vi "Measurement.vi"(0 "Position":T7(array[cluster]) {"Z" format="%.1f"; "Y" format="%.1f"; "X" format="%.1f"}, 1 "setup":T8=enum."Show Setup", 2 "Post Process":T5, 4 "File":T9, 5 "Results file":path, 7 "Raw data file":path, 11 "Setup filename":string) -> (14 "2nd plot":cluster{"Xo":dbl, "Delta X":dbl, dbl[]}[](graph), 19 "Status Out":T4)   [LabVIEW 2011]
uses:
  Anemometry Sub Vis/Controls/Save_Data.ctl
  Anemometry Sub Vis/Controls/Setup.ctl
  Anemometry Sub Vis/Controls/Graph_Type.ctl
  Anemometry Sub Vis/Controls/Post_Process.ctl
  Anemometry Sub Vis/Gen Trav/Multi_Run_Status.ctl
  Anemometry Sub Vis/Controls/Board_Types.ctl
  Anemometry Sub Vis/File/Setup_Filetype.ctl
  Anemometry Sub Vis/Controls/Block_start_and_end.ctl
  ADAM Client/Sub VIs/ADAM Controls/Traverse_Level_State.ctl
  Anemometry Sub Vis/Globals/Trav_pos_global.vi
  Anemometry Sub Vis/Globals/Meas_global.vi
  Anemometry Sub Vis/Acquisition/Data_Translation/DataTranslation_global.vi
  Anemometry Sub Vis/Acquisition/PWA/PWAtasksGLOBAL.vi
  Anemometry Sub Vis/Globals/Preference_global.vi
  Anemometry Sub Vis/Globals/LDA_meas_global_1.vi
  Anemometry Sub Vis/Globals/Dynamic_call_global.ph.vi
  Anemometry Sub Vis/Globals/LDA_meas_global_2.vi
  Anemometry Sub Vis/Globals/Plug_in_data_global.vi
panel:
  in  "PP next block":bool
  out "Pause message":string
  out "Statistics":string[][](table)
  in  "Tab Control":T1(tab)
  out "Measurement time (min)":dbl=6.0 format="%.2f"
  in  "No of bins":i32=80
  in  "Show Smoth":bool=TRUE
  in  "Second Graph":T3={"Plot 1"=2, "Plot 2"=1, "Save graph"=0, "Plot Type"=enum."Vel histogram"} {"Save graph" items=["Do not save plot", "Save plot"]; "Plot 2" items=["Nothing", "Mano (Pitot)", "RV (Uhw)", "RV (Kulite)"]; "Plot 1" items=["Nothing", "Mano (Pitot)", "RV (Uhw)", "RV (Kulite)"]}
  in  "First Graph":T3={"Plot 1"=1, "Plot 2"=2, "Save graph"=0, "Plot Type"=enum."Velocity trace"} {"Save graph" items=["Do not save plot", "Save plot"]; "Plot 2" items=["Nothing", "Mano (Pitot)", "RV (Uhw)", "RV (Kulite)"]; "Plot 1" items=["Nothing", "Mano (Pitot)", "RV (Uhw)", "RV (Kulite)"]}
  out "First plot":cluster{"Xo":dbl, "Delta X":dbl, dbl[]}[](graph)
  in  "Comments":string
  out "BSA Diagnostic info":string[][](table)
  out "uv":dbl[][](graph)=[[-0.041806189081711534, -0.046435429052714985, -0.04035660097427599, -0.042187605126076694, -0.042052555599004206]]
  out "u^4":dbl[][](graph)
  out "u^3":dbl[][](graph)
  out "u^2":dbl[][](graph)=[[0.09743628875280319, 0.10575821456272283, 0.10126262927293661, 0.09890442087602569, 0.1022948212436432]]
  out "U":dbl[][](graph)=[[0.8295029456391334, 0.8915896983798417, 0.8415763502225625, 0.8394746126219594, 0.8466062785395404]]
  in  "Block average display control":cluster{"Name":string, "Include":bool}[](array[cluster])=[{"Name"="FF (C)", "Include"=FALSE}]
  out "Array U":dbl[][](array[numeric]) format="%.2e"
  out "Array u^2":dbl[][](array[numeric]) format="%.2e"
  out "Actual Sampling freq":dbl=100.0 format="%.1f"
  in  "Desired Sampling freq (Hz)":dbl=100.0 format="%.1f"
  in  "Correlate?":T6(ring)
  out "Current Block No":i32=5
  in  "Pause":bool
  in  "No of Blocks":i32=5
  in  "stop":bool
  in  "No of samples":i32=1000 min=0 step=1
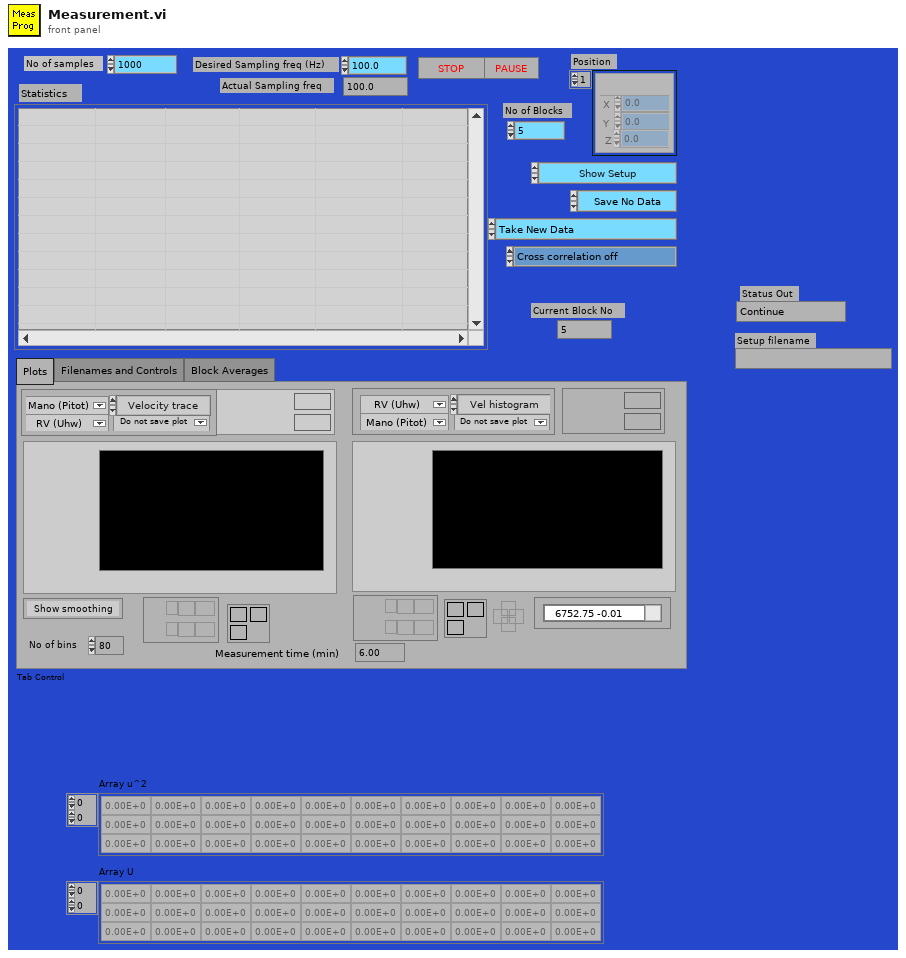
[diagram p1: front panel]
types:
  T1 = enum32{"Plots", "Filenames and Controls", "Block Averages"}
  T2 = typedef "Graph_Type.ctl" = enum16{"Show no graph", "Voltage trace", "Velocity trace", "Vel histogram", "Spectrum", "f.E(f) v Log f", "Auto-Corr"}
  T3 = cluster{"Plot 1":u16, "Plot 2":u16, "Save graph":u16, "Plot Type":T2}
  T4 = typedef "Multi_Run_Status.ctl" = enum16{"Continue", "Jump to Next Point", "Jump to Next Row", "Jump To Fall Back", "Terminate Run"}
  T5 = typedef "Post_Process.ctl" = enum16{"Take New Data", "Post Process Raw Data File"}
  T6 = enum16{"Cross correlation off", "Show correlation panel", "Correlate without activating panel"}
  T7 = cluster{"Name":string, "X":dbl, "Y":dbl, "Z":dbl}[]
  T8 = typedef "Setup.ctl" = enum16{"Run Program", "Show Setup", "Save Current Setup", "Setup Front Panel"}
  T9 = typedef "Save_Data.ctl" = enum16{"Save No Data", "Save Data"}
  T10 = enum32{"Bad", "Idle", "Run top level", "Running"}
  T11 = enum16{"Velocity", "Transit time", "Arrival time"}
  T12 = enum16{"Save no data", "Save data in new files", "Save data in existing files"}
  T13 = typedef "Board_Types.ctl" = enum16{"Simulate", "Local ADAM", "Server ADAM", "NI-DAQmx", "NI-DAQmxBase", "ADC488", "DT LV-link"}
  T14 = typedef "Setup_Filetype.ctl" = enum16{"Measurement Setups", "Calibration Setups", "General", "Results File Plotter Setups", "Speed Calib Tweaks"}
  T15 = typedef "Block_start_and_end.ctl" = cluster{"Started":dbl, "Ended":dbl, "Analogue Frequency Hz":dbl}
  T16 = typedef "Traverse_Level_State.ctl" = enum16{"Running", "Complete"}
  T17 = typedef "Traverse_cluster.ctl" = cluster{"Start X":dbl, "Start Y":dbl, "Start Z":dbl, "End X":dbl, "End Y":dbl, "End Z":dbl, "No. of pts.":i32, "Spacing":T18, "Filename":path, "Tunnel Speed":dbl, "Averaging time (min)":dbl, "Extra Commands":string, "Specific Arguments":string, "Emission Rate (l/min)":dbl, "Trace Gas Concentration (%)":dbl, "Density Ratio":string, "Comments":string, "Row No":i32, "Row Type Selector":T19, "Completion time":string, "Row Duration (mins)":dbl, "No. of Valid pts.":i32, "Meas Setup File":string}
  T18 = typedef "Spacing.ctl" = enum16{"Linear", "Log", "Gauss", "Specified", "N/A"}
  T19 = typedef "Multi_run_mode.ctl" = enum16{"Move Traverse Only", "Set Tunnel Speed Only", "Set Source Only", "Set Measurement Conditions", "Single Measurement", "Vertical Profile", "Lateral Profile", "Longitudinal Profile", "Explore Volume", "Multi-Axis Profile", "Auto Calibrate", "Meas Fast FID Bkgnd", "Check Beam Power", "Scanning Valve Measurement", "Run VI Named:", "Set ADAM Ch", "Wait (minutes)", "Send Message", "Synchronize With:", "Fall Back to this Row", "Turn Off Row Repeating", "Blank Row"}
  T20 = typedef "Analysis_info_cluster.ctl" = cluster{"Colour":u32, "Inst type":T21, "Inst name":string, "Symbol":string, "Code name":string, "Extra Info":string, "Inst Array":T22, "Index":i32, "Voltage Index":i32, "Extra Titles":string[], "Extra Values":string[]}
  T21 = typedef "Inst_type.ctl" = enum16{"Propeller anemometer", "Raw voltage", "Pressure Transducer", "Pitot-static tube", "Preston tube", "Hot wire", "Cross wire 1", "Cross wire 2", "Generic Linear", "Generic Polynomial", "Generic BackPoly", "Fast FID", "Thermocouple", "Cold wire", "Pulsed Wire", "LDA Vel", "LDA Tran time", "LDA Arr time"}
  T22 = typedef "Instrument_Array.ctl" = enum16{"PWA", "LDA", "Analogue"}
  T23 = enum16{"Velocity", "Transit time", "Arrival time"}[]
  T24 = typedef "BSA_Type.ctl" = enum16{"57N11", "BSA F60"}
  T25 = typedef "BSA_info_Cluster.ctl" = cluster{"GPIB Address":string, "No of Check Bytes":i32, "Extra Info":string, "COLOUR":u32, "Wavelength (nm)":dbl}
  T26 = typedef "Ch_and_Spans.ctl" = cluster{"high limit (10V)":sgl, "low limit (-10V)":sgl, "Ch No":i16, "Var name":string, "Use Latest Calib":bool}
  T27 = typedef "Velocity_cluster.ctl" = cluster{"Name":string, "U":dbl, "u^2":dbl, "u^3/(u^2)^(1.5)":dbl, "u^4/(u^2)^2 -3":dbl, "% u'/U":dbl, "Mean % Err":dbl, "u^4":dbl}
  T28 = typedef "Analysis_type_cluster.ctl" = cluster{"Analysis type":T29, "Indicies":i32[], "Name":string, "Inst Array":T22, "Info index":i32}
  T29 = typedef "Analysis_type_Enum.ctl" = enum16{"Slow Response", "Fast Response", "Weighted Fast Response", "Fast FID", "Weighted Fast FID", "Cross Wire", "Weighted Cross Wire", "Weighted LDA"}
  T30 = cluster{"Insts for plotting[0]":u16, "Insts for plotting[1]":u16}
  T31 = typedef "PWA_Data.ctl" = enum16{"No PWA Data", "One Ch PWA"}
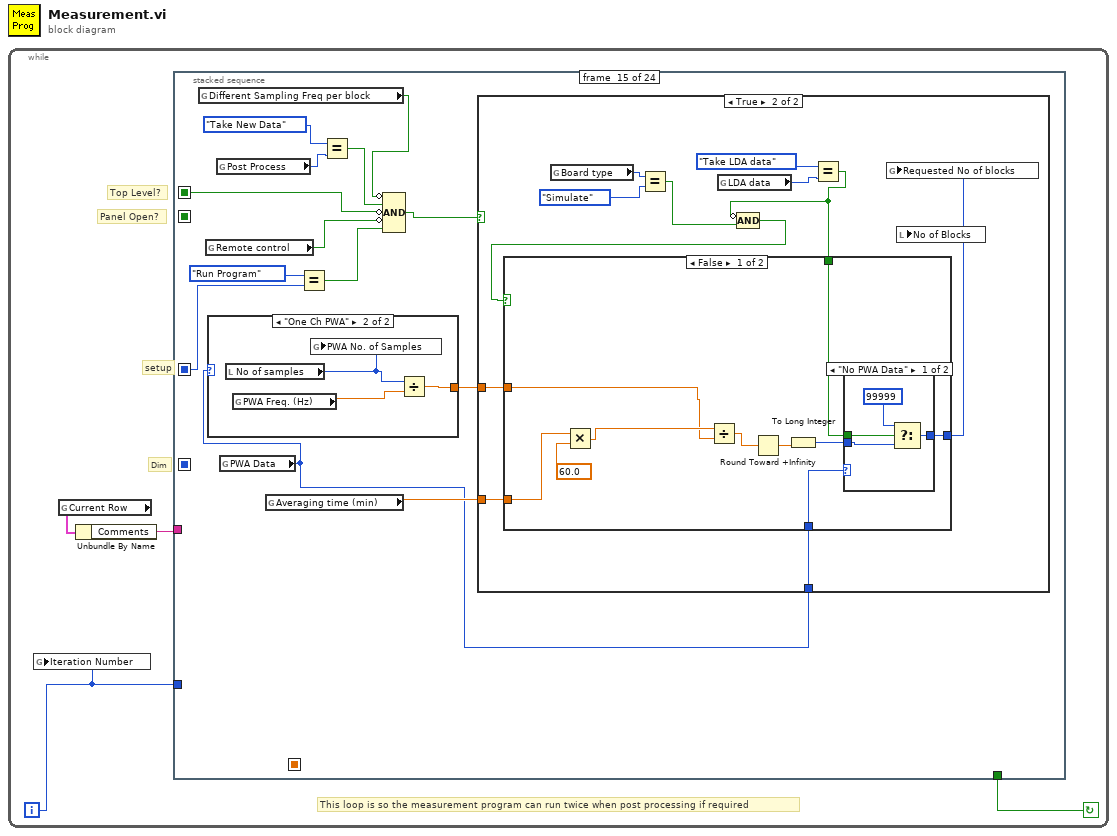
[diagram p0: block diagram]
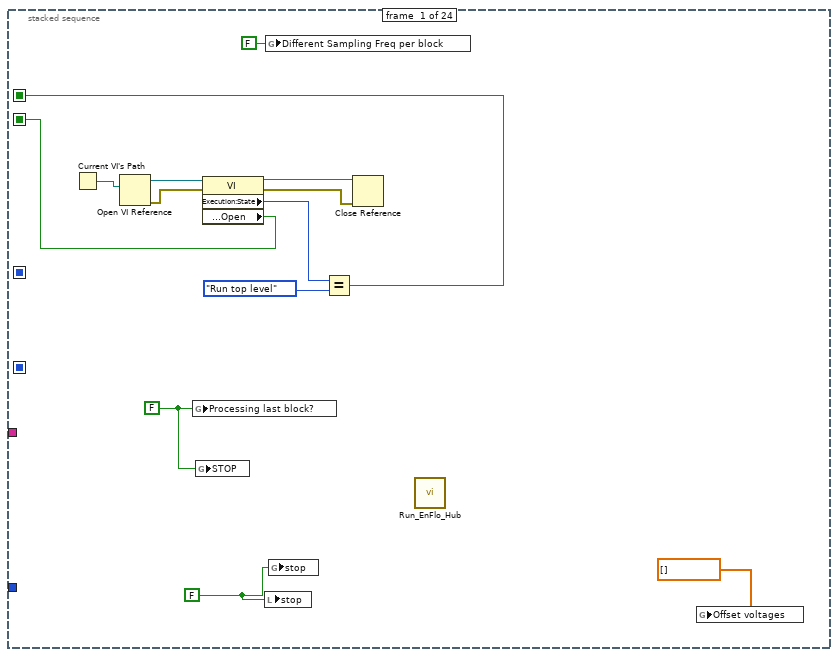
[diagram p2: hidden frame]
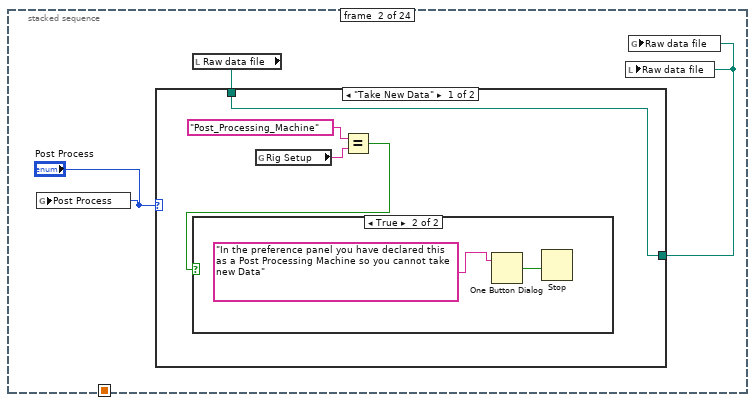
[diagram p3: hidden frame]
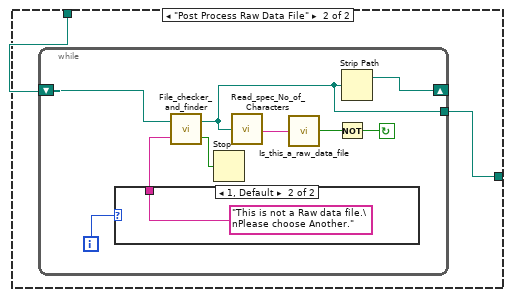
[diagram p5: hidden frame]
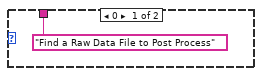
[diagram p6: hidden frame]
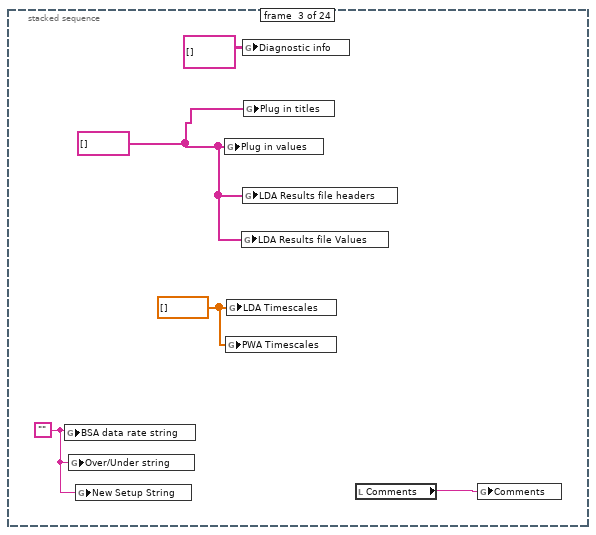
[diagram p7: hidden frame]
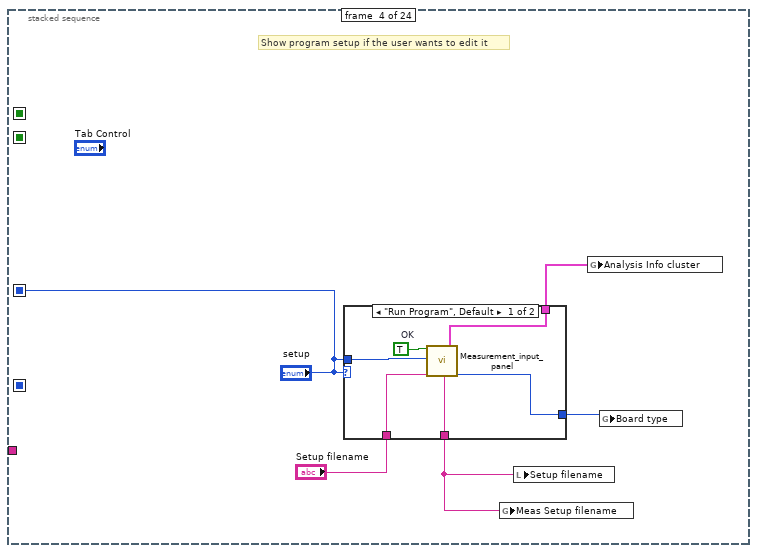
[diagram p8: hidden frame]
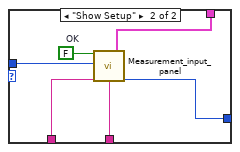
[diagram p9: hidden frame]
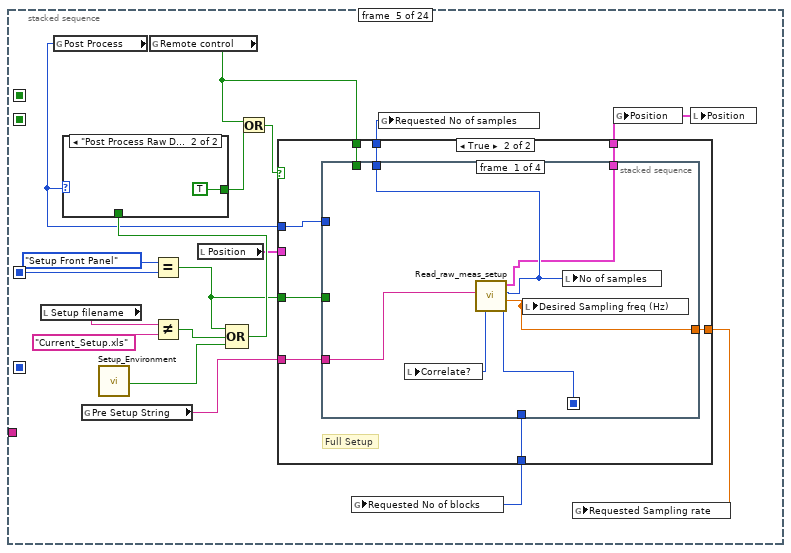
[diagram p10: hidden frame]
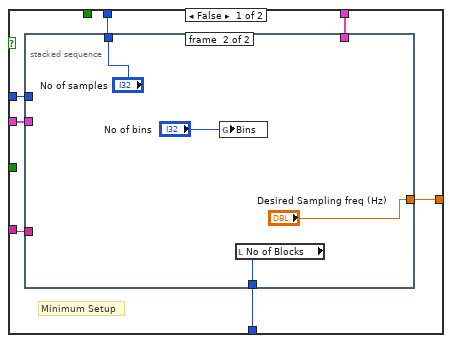
[diagram p12: hidden frame]
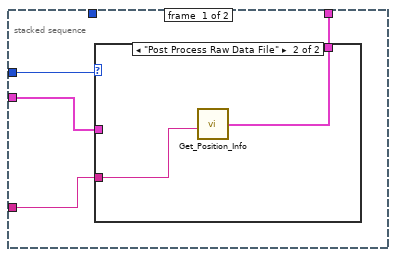
[diagram p13: hidden frame]
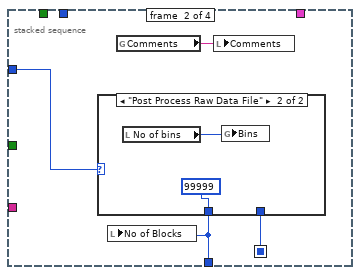
[diagram p15: hidden frame]
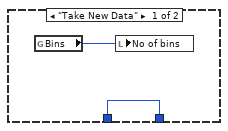
[diagram p16: hidden frame]
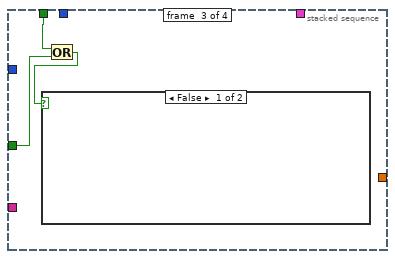
[diagram p17: hidden frame]
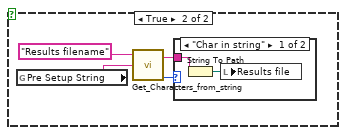
[diagram p18: hidden frame]
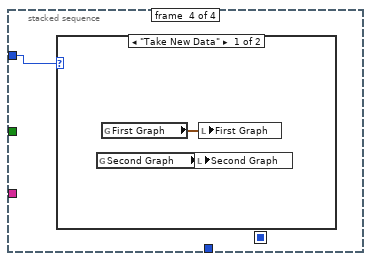
[diagram p20: hidden frame]
diagram:
  n1 = while {
    i -> [w1]
    stop <- w2 continue-if-true
    # "This loop is so the measurement program can run twice when post processing if required"
    # "Panel Open?"
    # "Top Level?"
    # "setup"
    # "Dim"
    n2 = global write "Meas_global.vi" "Iteration Number"(w1) -> ()
    n3 = global read "Trav_pos_global.vi" "Current Row"() -> (w3:T17)
    n4 = Unbundle By Name(w3) -> ("Comments"=w4:string)
    n5 = stacked-sequence {
      seq-local: [_ _ _ _ _ _ _ _ w187 _ _ _ _ _ _ _ _ _ _ _ _ _ _ _] -> [_ _ _ _ _ _ _ _ _ _ _ _ _ _ _ _ _ w626 _ _ _ _ _ _]
      seq-local: [_ _ _ "setup" _ _ _ _ _ _ _ _ _ _ _ _ _ _ _ _ _ _ _ _] -> [_ _ _ _ w71 _ _ _ w179 w264 _ _ _ _ w524 w564 w571 w627 w935 w1011 w1039 _ _ w1114]
      seq-local: [_ _ _ _ _ _ _ _ _ _ _ _ _ _ _ _ w567 _ _ _ _ _ _ _] -> [_ _ _ _ _ _ _ _ _ _ _ _ _ _ _ _ _ w625 w918 _ _ _ _ _]
      seq-local: [w7 _ _ _ _ _ _ _ _ _ _ _ _ _ _ _ _ _ _ _ _ _ _ _] -> [_ _ _ _ _ _ _ _ _ w244 _ _ _ _ w520 _ _ w624 _ _ _ _ _ _]
      seq-local: [w6 _ _ _ _ _ _ _ _ _ _ _ _ _ _ _ _ _ _ _ _ _ _ _] -> [_ _ _ _ _ _ _ _ _ _ _ _ w363 _ _ _ _ _ _ _ _ _ _ _]
      tunnel: w4 -> [_ _ _ _ _ _ _ w172 _ _ _ _ _ _ _ _ _ _ _ _ _ _ w1082 _]
      tunnel: w1 -> [_ _ _ _ _ _ _ _ _ _ _ _ _ _ _ _ _ _ _ _ _ _ w1077 _]
      tunnel: [_ _ _ _ _ _ _ _ _ _ _ _ _ _ _ _ _ _ _ _ _ _ w1076 _] -> w2
      frame #0 {
        w15 = FALSE ("Processing last block?")
        w16 = FALSE ("stop")
        n6 = Current VI's Path() -> (path=w8:path)
        n7 = Open VI Reference(vi path=w8) -> (vi reference=w9:refnum<vi>, error out=w10:errorcluster)  [unwired: 1 in, 4 out]
        n8 = global write "Meas_global.vi" "Processing last block?"(w15) -> ()
        n9 = global write "PWAtasksGLOBAL.vi" "STOP"(w15) -> ()
        n10 = property class="VI"(reference=w9, error in=w10) -> (reference out=w11:refnum<vi>, error out=w12:errorcluster, "Execution:State"=w13:T10, "Front Panel.Open"=w6:bool)
        n11 = local write "stop"(w16) -> ()
        n12 = global write "DataTranslation_global.vi" "Different Sampling Freq per block"(FALSE ("Different Sampling Freq per block")) -> ()
        n13 = global write "Meas_global.vi" "stop"(w16) -> ()
        n14 = Equal?(x=w13, y=T10."Run top level" ("Exec.State")) -> (x = y?=w7:bool)
        n15 = Close Reference(reference=w11, error in (no error)=w12) -> ()  [unwired: 1 out]
        n16 = call "Run_EnFlo_Hub.vi"() -> ()  [unwired: 8 out]
        n17 = global write "Meas_global.vi" "Offset voltages"(dbl[] [] ("Offset voltages used")) -> ()
      }
      frame #1 {
        n18 = global write "Meas_global.vi" "Post Process"("Post Process") -> ()
        n19 = local read "Raw data file"() -> (w20:path)
        n20 = case shown="\"Take New Data\"" "Post Process" {
          tunnel: [w24 w28] -> w19
          tunnel: w20 -> [w24 w27]
          frame "Take New Data" {
            n21 = global read "Preference_global.vi" "Rig Setup"() -> (w23:string)
            n22 = Equal?(x="Post_Processing_Machine" ("Rig Setup"), y=w23) -> (x = y?=w21:bool)
            n23 = case shown="True" w21 {
              frame False {
              }
              frame True {
                n24 = One Button Dialog(message="In the preference panel you have declared this as a Post Processing Machine so you cannot take new Data") -> (true=w25:bool)  [unwired: 1 in]
                n25 = Stop(stop? (T)=w25) -> ()
              }
            }
          }
          frame "Post Process Raw Data File" {
            n26 = while {
              tunnel: [w30] -> w28
              shift-left: w27 -> [w32]
              shift-right: [w31] -> _
              i -> [w33]
              stop <- w34 continue-if-true
              n27 = case shown="1, Default" w33 {
                tunnel: ["Find a Raw Data File to Post Process" ("Promp if not found") "This is not a Raw data file.\nPlease choose Another." ("Promp if not found")] -> w37
                frame 0 {
                }
                frame 1, Default {
                }
              }
              n28 = call "File_checker_and_finder.vi"("Promp if not found"=w37, "Filename In"=w32) -> ("cancelled"=w29:bool, "Filename Out"=w30:path)
              n29 = Stop(stop? (T)=w29) -> ()
              n30 = call "Read_spec_No_of_Characters.vi"("Filename"=w30) -> ("character string"=w36:string)  [unwired: 1 out]
              n31 = call "Is_this_a_raw_data_file.vi"("character string"=w36) -> ("Raw Dat File?"=w35:bool)  [unwired: 2 out]
              n32 = Not(x=w35) -> (.not. x?=w34:bool)
              n33 = Strip Path(path=w30) -> (stripped path=w31:path)  [unwired: 1 out]
            }
          }
        }
        n34 = local write "Raw data file"(w19) -> ()
        n35 = global write "Meas_global.vi" "Raw data file"(w19) -> ()
      }
      frame #2 {
        w42 = dbl[] [] ("LDA Timescales")
        w41 = string[] [] ("Plug in values")
        w44 = ""
        n36 = global write "Meas_global.vi" "BSA data rate string"(w44) -> ()
        n37 = global write "Meas_global.vi" "Over/Under string"(w44) -> ()
        n38 = global write "Meas_global.vi" "New Setup String"(w44) -> ()
        n39 = global write "Dynamic_call_global.ph.vi" "Plug in values"(w41) -> ()
        n40 = global write "PWAtasksGLOBAL.vi" "PWA Timescales"(w42) -> ()
        n41 = global write "LDA_meas_global_1.vi" "LDA Timescales"(w42) -> ()
        n42 = global write "LDA_meas_global_1.vi" "LDA Results file Values"(w41) -> ()
        n43 = global write "Meas_global.vi" "Diagnostic info"(string[][] [] ("Diagnostic info")) -> ()
        n44 = global write "LDA_meas_global_1.vi" "LDA Results file headers"(w41) -> ()
        n45 = global write "Dynamic_call_global.ph.vi" "Plug in titles"(w41) -> ()
        n46 = local read "Comments"() -> (w43:string)
        n47 = global write "Meas_global.vi" "Comments"(w43) -> ()
      }
      frame #3 {
        # "Show program setup if the user wants to edit it"
        n48 = case shown="\"Run Program\", Default" "setup" {
          tunnel: [w54 w60] -> w49
          tunnel: [w53 w59] -> w48
          tunnel: "Setup filename" -> [w52 w58]
          tunnel: [w51 w57] -> w45
          tunnel: "setup" -> [w50 w56]
          frame "Run Program", Default {
            w55 = TRUE  # OK
            n49 = call "Measurement_input_panel.vi"("OK"=w55, "setup"=w50, "Setup filename"=w52) -> ("Setup filename out"=w51:string, "Analysis Info cluster"=w54:T20[], "Board type"=w53:T13)  [unwired: 14 out]
          }
          frame "Show Setup" {
            w61 = FALSE  # OK
            n50 = call "Measurement_input_panel.vi"("OK"=w61, "setup"=w56, "Setup filename"=w58) -> ("Setup filename out"=w57:string, "Analysis Info cluster"=w60:T20[], "Board type"=w59:T13)  [unwired: 14 out]
          }
        }
        n51 = global write "Meas_global.vi" "Meas Setup filename"(w45) -> ()
        n52 = local write "Setup filename"(w45) -> ()
        n53 = global write "Meas_global.vi" "Analysis Info cluster"(w49) -> ()
        n54 = global write "Meas_global.vi" "Board type"(w48) -> ()
      }
      frame #4 {
        n55 = local read "Setup filename"() -> (w75:string)
        n56 = global read "Meas_global.vi" "Post Process"() -> (w70:T5)
        n57 = global read "Meas_global.vi" "Pre Setup String"() -> (w66:string)
        n58 = call "Setup_Environment.vi"() -> ("First Time"=w67:bool)  [unwired: 1 in]
        n59 = global read "Meas_global.vi" "Remote control"() -> (w63:bool)
        n60 = Equal?(x=Setup."Setup Front Panel" ("setup"), y=w71) -> (x = y?=w62:bool)
        n61 = Not Equal?(x=w75, y="Current_Setup.xls" ("Setup filename")) -> (x != y?=w73:bool)
        n62 = local read "Position"() -> (w64:T7)
        n63 = Compound Arithmetic op=OR(w62, w73, w67) -> (w72:bool)
        n64 = case shown="\"Post Process Raw Data File\"" w70 {
          tunnel: [w80 TRUE] -> w79
          tunnel: w72 -> [w80 _]
          frame "Take New Data" {
          }
          frame "Post Process Raw Data File" {
          }
        }
        n65 = Or(x=w63, y=w79) -> (x .or. y?=w78:bool)
        n66 = case shown="True" w78 {
          tunnel: w70 -> [w84 w107]
          tunnel: [w88 w106] -> w68
          tunnel: [w87 w101] -> w77
          tunnel: [w86 w105] -> w76
          tunnel: [w85 w104] -> w65
          tunnel: w66 -> [w83 w103]
          tunnel: w64 -> [w82 _]
          tunnel: w63 -> [_ w102]
          tunnel: w62 -> [_ w100]
          frame False {
            # "Minimum Setup"
            n67 = stacked-sequence {
              tunnel: [_ "Desired Sampling freq (Hz)"] -> w88
              tunnel: [_ w98] -> w87
              tunnel: [_ "No of samples"] -> w86
              tunnel: [w91 _] -> w85
              tunnel: w84 -> [w92 _]
              tunnel: w83 -> [w90 _]
              tunnel: w82 -> [w89 _]
              frame #0 {
                n68 = case shown="\"Post Process Raw Data File\"" w92 {
                  tunnel: [w93 w94] -> w91
                  tunnel: w89 -> [w93 _]
                  tunnel: w90 -> [_ w95]
                  frame "Take New Data" {
                  }
                  frame "Post Process Raw Data File" {
                    n69 = call "Get_Position_Info.vi"("Input string"=w95) -> ("Position"=w94:T7)
                  }
                }
              }
              frame #1 {
                n70 = global write "Meas_global.vi" "Bins"("No of bins") -> ()
                n71 = local read "No of Blocks"() -> (w98:i32)
              }
            }
          }
          frame True {
            # "Full Setup"
            n72 = stacked-sequence {
              seq-local: [w110 _ _ _] -> [_ w115 _ _]
              tunnel: w107 -> [_ w116 _ w131]
              tunnel: [w113 _ _ _] -> w106
              tunnel: [w112 _ _ _] -> w105
              tunnel: [w108 _ _ _] -> w104
              tunnel: w103 -> [w111 _ _ _]
              tunnel: w102 -> [_ _ w124 _]
              tunnel: [_ w114 _ _] -> w101
              tunnel: w100 -> [_ _ w123 _]
              frame #0 {
                n73 = call "Read_raw_meas_setup.vi"("Setup file string"=w111) -> ("No of Blocks"=w110:i32, "Sampling freq (Hz)"=w113:dbl, "No of samples"=w112:i32, "Position"=w108:T7, "Correlate?"=w109:T6)  [unwired: 4 out]
                n74 = local write "Correlate?"(w109) -> ()
                n75 = local write "Desired Sampling freq (Hz)"(w113) -> ()
                n76 = local write "No of samples"(w112) -> ()
              }
              frame #1 {
                n77 = case shown="\"Post Process Raw Data File\"" w116 {
                  tunnel: [w119 99999 ("No of Blocks")] -> w114
                  tunnel: w115 -> [w119 _]
                  frame "Take New Data" {
                    n78 = global read "Meas_global.vi" "Bins"() -> (w118:i32)
                    n79 = local write "No of bins"(w118) -> ()
                  }
                  frame "Post Process Raw Data File" {
                    n80 = local read "No of bins"() -> (w120:i32)
                    n81 = global write "Meas_global.vi" "Bins"(w120) -> ()
                  }
                }
                n82 = local write "No of Blocks"(w114) -> ()
                n83 = global read "Meas_global.vi" "Comments"() -> (w117:string)
                n84 = local write "Comments"(w117) -> ()
              }
              frame #2 {
                n85 = Or(x=w124, y=w123) -> (x .or. y?=w122:bool)
                n86 = case shown="False" w122 {
                  frame False {
                  }
                  frame True {
                    n87 = global read "Meas_global.vi" "Pre Setup String"() -> (w125:string)
                    n88 = call "Get_Characters_from_string.vi"("Input string"=w125, "Variable name"="Results filename") -> ("Status"=w128:enum16{"Char in string", "Char not in string"}, "Value"=w127:string)  [unwired: 1 in]
                    n89 = case shown="\"Char in string\"" w128 {
                      tunnel: w127 -> [w130 _]
                      frame "Char in string" {
                        n90 = String To Path(string=w130) -> (path=w129:path)
                        n91 = local write "Results file"(w129) -> ()
                      }
                      frame "Char not in string" {
                      }
                    }
                  }
                }
              }
              frame #3 {
                n92 = case shown="\"Take New Data\"" w131 {
                  frame "Take New Data" {
                    n93 = global read "Meas_global.vi" "Second Graph"() -> (w132:T3)
                    n94 = global read "Meas_global.vi" "First Graph"() -> (w133:T3)
                    n95 = local write "Second Graph"(w132) -> ()
                    n96 = local write "First Graph"(w133) -> ()
                  }
                  frame "Post Process Raw Data File" {
                  }
                }
              }
            }
          }
        }
        n97 = global write "Meas_global.vi" "Requested No of blocks"(w77) -> ()
        n98 = global write "Meas_global.vi" "Requested No of samples"(w76) -> ()
        n99 = global write "Meas_global.vi" "Requested Sampling rate"(w68) -> ()
        n100 = global write "Meas_global.vi" "Position"(w65) -> ()
        n101 = local write "Position"(w65) -> ()
      }
      frame #5 {
        n102 = global read "Meas_global.vi" "Post Process"() -> (w134:T5)
        n103 = case shown="\"Post Process Raw Data File\"" w134 {
          tunnel: [w137 w138] -> w135
          frame "Take New Data" {
            n104 = Get Date/Time In Seconds() -> (seconds since 1Jan1904=w136:timestamp)
            n105 = To Double Precision Float(number=w136) -> (double precision float=w137:dbl)
          }
          frame "Post Process Raw Data File" {
            n106 = global read "Meas_global.vi" "Pre Setup String"() -> (w141:string)
            n107 = call "Get_Characters_from_string.vi"("Input string"=w141, "Variable name"="Seconds since 1/1/04") -> ("Value"=w139:string)  [unwired: 1 in, 1 out]
            n108 = call "String_2_Number.vi"("Value"=w139) -> ("Numeric"=w138:dbl)
          }
        }
        n109 = global write "Meas_global.vi" "Time Data was Aquired"(w135) -> ()
      }
      frame #6 {
        n110 = global read "Dynamic_call_global.ph.vi" "Initial Plug Ins"() -> (w143:string[])
        n111 = global read "Dynamic_call_global.ph.vi" "Initial Plug Ins Extra"() -> (w144:string[])
        n112 = Build Array (concatenate)(w144, w143) -> (w142:string[])
        n113 = Array Size(array=w142) -> (size(s)=w146:i32)
        n114 = Greater Than 0?(x=w146) -> (x > 0?=w145:bool)
        n115 = case shown="True" w145 {
          tunnel: w142 -> [_ w147]
          frame False {
          }
          frame True {
            n116 = stacked-sequence {
              tunnel: w147 -> [w149 _]
              frame #0 {
                n117 = global read "Meas_global.vi" "Post Process"() -> (w151:T5)
                n118 = call "Plug_in_Directories.vi"() -> ("Initial"=w148:path)  [unwired: 3 out]
                n119 = Equal?(x=w151, y=Post_Process."Post Process Raw Data File" ("Post Process")) -> (x = y?=w150:bool)
                n120 = for {
                  tunnel: w150 -> [w157]
                  tunnel: w149 -> [w154] mode=indexing
                  tunnel: w148 -> [w153]
                  w164 = FALSE  # Dialog Box (T)
                  n121 = Build Path(base path=w153, name or relative path=w154) -> (appended path=w155:path)
                  n122 = Open VI Reference(vi path=w155) -> (vi reference=w162:refnum<vi>, error out=w161:errorcluster)  [unwired: 2 in, 3 out]
                  n123 = property class="VI"(reference=w162, error in=w161, "Front Panel Window:Open"=TRUE ("Wait until done")) -> (reference out=w160:refnum<vi>, error out=w159:errorcluster)
                  n124 = invoke class="VI" method="Run VI"(reference=w160, error in=w159, "Wait until done"=w157, "Auto Dispose Ref"=FALSE) -> (reference out=w167:refnum<vi>, error out=w166:errorcluster)  [unwired: 1 in, 3 out]
                  n125 = Close Reference(reference=w167, error in (no error)=w166) -> (error out=w165:errorcluster)
                  n126 = call "EnFlo_Error_Handler.vi"("error in (no error)"=w165, "Error Type"="Launching Initial Plug In", "Dialog Box (T)"=w164) -> ()  [unwired: 3 out]
                }
              }
              frame #1 {
                n127 = global read "Meas_global.vi" "Requested No of blocks"() -> (w169:i32)
                n128 = global read "Meas_global.vi" "Comments"() -> (w168:string)
                n129 = local write "Comments"(w168) -> ()
                n130 = local write "No of Blocks"(w169) -> ()
              }
            }
          }
        }
      }
      frame #7 {
        n131 = local read "Comments"() -> (w173:string)
        n132 = Concatenate Strings(w172, w173) -> (w171:string)
        n133 = call "Text_without_format.vi"("Input string"=w171) -> ("Output string"=w170:string)
        n134 = local write "Comments"(w170) -> ()
        n135 = global write "Meas_global.vi" "Comments"(w170) -> ()
      }
      frame #8 {
        n136 = global read "Meas_global.vi" "dimensions"() -> (w187:enum16{"1D", "2D"})
        n137 = global read "Meas_global.vi" "Post Process"() -> (w186:T5)
        n138 = global read "Meas_global.vi" "LDA data"() -> (w184:enum16{"No LDA data", "Take LDA data"})
        n139 = Equal?(x=Setup."Run Program" ("setup"), y=w179) -> (x = y?=w182:bool)
        n140 = Equal?(x=w179, y=Setup."Show Setup" ("setup")) -> (x = y?=w174:bool)
        n141 = Equal?(x=w184, y=enum16{"No LDA data", "Take LDA data"}."Take LDA data" ("LDA data")) -> (x = y?=w177:bool)
        n142 = Or(x=w182, y=w174) -> (x .or. y?=w176:bool)
        n143 = Equal?(x=w186, y=Post_Process."Take New Data" ("Post Process")) -> (x = y?=w178:bool)
        n144 = Compound Arithmetic op=AND(w176, w177, w178) -> (w175:bool)
        n145 = case shown="True" w175 {
          tunnel: w187 -> [_ w196]
          tunnel: w179 -> [_ w195]
          tunnel: w174 -> [_ w193]
          frame False {
            n146 = global write "LDA_meas_global_1.vi" "Number of measured quantities"(3 ("Number of measured quantities")) -> ()
            n147 = Build Array(T11."Velocity", T11."Transit time", T11."Arrival time") -> (w188:T23)
            n148 = global write "LDA_meas_global_2.vi" "data type"(w188) -> ()
            n149 = global write "LDA_meas_global_1.vi" "data type"(w188) -> ()
          }
          frame True {
            n150 = global read "LDA_meas_global_1.vi" "BSA Type"() -> (w194:T24)
            n151 = case shown="\"BSA F60\"" w194 {
              tunnel: w196 -> [w198 _]
              tunnel: w195 -> [w197 _]
              tunnel: w193 -> [_ w234]
              frame "57N11" {
                n152 = stacked-sequence {
                  tunnel: w198 -> [w201 w227]
                  tunnel: w197 -> [w200 _]
                  frame #0 {
                    n153 = global read "Meas_global.vi" "Remote control"() -> (w199:bool)
                    n154 = case shown="\"2D\"" w201 {
                      tunnel: w200 -> [w203 w216]
                      tunnel: w199 -> [w202 w215]
                      frame "2D" {
                        n155 = while {
                          tunnel: w202 -> [w204]
                          tunnel: w203 -> [w205]
                          stop <- w206 continue-if-true
                          n156 = stacked-sequence {
                            tunnel: [_ _ w212] -> w206
                            tunnel: w205 -> [w207 w209 _]
                            tunnel: w204 -> [_ _ w211]
                            frame #0 {
                              w208 = "1"  # BSA Number
                              n157 = call "Control_BSA_setup.vi"("setup"=w207, "BSA number"=w208) -> ()  [unwired: 14 out]
                            }
                            frame #1 {
                              w210 = "2"  # BSA Number
                              n158 = call "Control_BSA_setup.vi"("setup"=w209, "BSA number"=w210) -> ()  [unwired: 14 out]
                            }
                            frame #2 {
                              n159 = case shown="False" w211 {
                                tunnel: [w213 FALSE ("ok")] -> w212
                                frame False {
                                n160 = call "BSA_setup_check.vi"() -> ("ok"=w213:bool)
                                }
                                frame True {
                                }
                              }
                            }
                          }
                        }
                      }
                      frame "1D" {
                        n161 = stacked-sequence {
                          tunnel: w216 -> [w217 _]
                          tunnel: w215 -> [_ _]
                          frame #0 {
                            w218 = "1"  # BSA Number
                            n162 = call "Control_BSA_setup.vi"("setup"=w217, "BSA number"=w218) -> ()  [unwired: 14 out]
                          }
                          frame #1 {
                            n163 = global read "LDA_meas_global_2.vi" "BSA2 info"() -> (w219:T25)
                            n164 = Unbundle By Name(w219) -> ("GPIB Address"=w220:string)
                            n165 = call "Set_BSA_Coincidence.vi"("GPIB address"=w220, "Set Coincidence"=enum16{"Slave", "Master", "Private"}."Slave") -> ()  [unwired: 1 in, 5 out]
                          }
                        }
                      }
                    }
                  }
                  frame #1 {
                    n166 = global read "Meas_global.vi" "Remote control"() -> (w225:bool)
                    n167 = Equal?(x=w227, y=enum16{"1D", "2D"}."2D" ("dimensions")) -> (x = y?=w223:bool)
                    n168 = Not(x=w225) -> (.not. x?=w224:bool)
                    n169 = And(x=w224, y=w223) -> (x .and. y?=w222:bool)
                    n170 = case shown="True" w222 {
                      frame False {
                      }
                      frame True {
                        n171 = global read "LDA_meas_global_1.vi" "BSA1 info"() -> (w229:T25)
                        n172 = global read "LDA_meas_global_2.vi" "BSA2 info"() -> (w230:T25)
                        n173 = Build Array(w229, w230) -> (w228:T25[])
                        n174 = for {
                          tunnel: w228 -> [w232] mode=indexing
                          n175 = Unbundle By Name(w232) -> ("GPIB Address"=w231:string)
                          n176 = call "Set_BSA_Coincidence.vi"("GPIB address"=w231, "Set Coincidence"=enum16{"Slave", "Master", "Private"}."Master") -> ()  [unwired: 1 in, 5 out]
                        }
                      }
                    }
                  }
                }
              }
              frame "BSA F60" {
                n177 = disable-structure shown="TARGET_TYPE==Windows" {
                  disable-tunnel: w234 -> [_ w235]
                  frame condition #0 (active) {
                  }
                  frame condition #1 {
                    n178 = while {
                      tunnel: w235 -> [w238]
                      stop <- w236 continue-if-true
                      n179 = call "Edit_BSA_IP.vi"("Show Panel"=w238) -> ("Run LDA Diagnostic Out"=w237:bool)  [unwired: 2 out]
                      n180 = case shown="False" w237 {
                        tunnel: [FALSE w240] -> w236
                        frame False {
                        }
                        frame True {
                          n181 = call "F60_Diagnostic.vi"() -> ("Edit BSA Setup Out"=w240:bool)  [unwired: 11 in]
                        }
                      }
                    }
                  }
                }
              }
            }
          }
        }
      }
      frame #9 {
        w249 = Save_Data."Save No Data" ("File")
        w265 = Post_Process."Take New Data"  # Post Process
        n182 = global read "Trav_pos_global.vi" "Meas Setup Number"() -> (w245:i32)
        n183 = Not Equal?(x=Setup."Run Program" ("setup"), y=w264) -> (x != y?=w250:bool)
        n184 = call "Current_Filepath.vi"("Filename in"="Results file", "Data Type"="Results") -> ("Filename Out"=w243:path)  [unwired: 1 out]
        n185 = global read "Meas_global.vi" "Remote control"() -> (w261:bool)
        n186 = global read "Meas_global.vi" "Post Process"() -> (w252:T5)
        n187 = Equal?(x="File", y=w249) -> (x = y?=w259:bool)
        n188 = case shown="1, Default" w245 {
          tunnel: [w268 w270] -> w246
          tunnel: w243 -> [w268 w277]
          tunnel: w245 -> [_ w278]
          frame 0 {
          }
          frame 1, Default {
            n189 = Add(x=96, y=w278) -> (x+y=w280:i32)
            n190 = Build Array(w280) -> (w281:i32[])
            n191 = Strip Path(path=w277) -> (stripped path=w271:path, name=w276:string)
            n192 = Byte Array To String(unsigned byte array=w281) -> (string=w274:string)
            n193 = call "Add_filename_suffix.vi"("Filename"=w276) -> ("Original Suffix"=w273:string, "Base name"=w275:string)  [unwired: 1 in, 2 out]
            n194 = Format Into String(format string="%s_%s%s", w275, w274, w273) -> (resulting string=w272:string)  [unwired: 2 in, 1 out]
            n195 = Build Path(base path=w271, name or relative path=w272) -> (appended path=w270:path)
          }
        }
        n196 = Equal?(x=w252, y=w265) -> (x = y?=w251:bool)
        n197 = And(x=w261, y=w251) -> (x .and. y?=w257:bool)
        n198 = Compound Arithmetic op=AND(w259, invert w261, w251, invert w250) -> (w260:bool)
        n199 = while {
          shift-left: _ -> [w286]
          shift-right: [w283] -> _
          tunnel: "File" -> [w284]
          tunnel: [w287] -> w258
          tunnel: w260 -> [w283]
          stop <- FALSE continue-if-true
          n200 = Compound Arithmetic op=AND(w283, invert w286) -> (w285:bool)
          n201 = case shown="True" w285 {
            tunnel: [w288 w291] -> w287
            tunnel: w284 -> [w288 _]
            frame False {
            }
            frame True {
              n202 = Two Button Dialog(message="Do you wish to save the data?", 1:"Save Data" ("F button name (\"Cancel\")"), 2:"Save No Data" ("T button name (\"OK\")")) -> (T button?=w292:bool)
              n203 = Select(t=Save_Data."Save No Data" ("File"), s=w292, f=Save_Data."Save Data" ("File")) -> (s? t:f=w291:T9)
            }
          }
        }
        n204 = Equal?(x=w249, y=w258) -> (x = y?=w248:bool)
        n205 = Or(x=w248, y=w250) -> (x .or. y?=w263:bool)
        n206 = case shown="False" w263 {
          tunnel: w246 -> [w307 w315]
          tunnel: [w306 w315] -> w266
          tunnel: "Raw data file" -> [w305 w316]
          tunnel: [w300 w316] -> w255
          tunnel: w264 -> [w304 _]
          tunnel: w258 -> [w303 _]
          tunnel: [w301 T12."Save no data" ("File output")] -> w253
          tunnel: [w302 w313] -> w247
          tunnel: w257 -> [_ w310]
          tunnel: w250 -> [_ w309]
          tunnel: w244 -> [w299 _]
          frame False {
            n207 = call "File_setup.vi"("Measurement is top level?"=w299, "Results file"=w307, "Raw data file"=w305, "setup"=w304, "File"=w303) -> ("Results file output"=w306:path, "Raw data file output"=w300:path, "Raw data option"=w302:enum16{"Save raw data", "Raw data not saved"}, "File output"=w301:T12)
          }
          frame True {
            w311 = enum16{"Save raw data", "Raw data not saved"}."Raw data not saved"  # Raw data option
            n208 = global read "Meas_global.vi" "Raw data option"() -> (w312:enum16{"Save raw data", "Raw data not saved"})
            n209 = Compound Arithmetic op=AND(w310, invert w309) -> (w308:bool)
            n210 = Select(t=w312, s=w308, f=w311) -> (s? t:f=w313:enum16{"Save raw data", "Raw data not saved"})
          }
        }
        n211 = case shown="\"Save raw data\"" w247 {
          tunnel: w255 -> [w296 w298]
          tunnel: [w296 w297] -> w254
          frame "Raw data not saved" {
          }
          frame "Save raw data" {
            n212 = call "Find_Unique_Filename.vi"("Path In"=w298) -> ("Unique Path Out"=w297:path)  [unwired: 1 in, 1 out]
          }
        }
        n213 = local write "Results file"(w266) -> ()
        n214 = global write "Meas_global.vi" "Results file"(w266) -> ()
        n215 = global write "Meas_global.vi" "Raw data option"(w247) -> ()
        n216 = global write "Meas_global.vi" "File"(w253) -> ()
        n217 = global write "Meas_global.vi" "Raw data file"(w254) -> ()
        n218 = local write "Raw data file"(w254) -> ()
        n219 = local write "File"(w258) -> ()
      }
      frame #10 {
        n220 = global read "Meas_global.vi" "Ch & spans"() -> (w317:T26[])
        n221 = local read "Block average display control"() -> (w322:cluster{"Name":string, "Include":bool}[])
        n222 = global read "Meas_global.vi" "Velocity Cluster Array"() -> (w321:T27[])
        n223 = global write "Meas_global.vi" "Ch & spans + mod limits"(w317) -> ()
        n224 = global read "Meas_global.vi" "Analysis Info cluster"() -> (w327:T20[])
        n225 = call "Determine_Meas_Analysis.vi"("Analogue Channels"=w327) -> ("Analysis Info Cluster"=w324:T20[], "Analysis Type Array"=w326:T28[])
        n226 = for {
          tunnel: w324 -> [w337] mode=indexing
          tunnel: w322 -> [w336]
          tunnel: w321 -> [w334]
          tunnel: [w328] -> w320 mode=indexing
          tunnel: [w331] -> w319 mode=indexing
          tunnel: [w330] -> w318 mode=indexing
          i -> [w335]
          w329 = nan ("Mean % Err")
          n227 = Unbundle By Name(w337) -> ("Inst name"=w328:string)
          n228 = Index Array(array=w334, index=w335) -> (element=w333:T27)
          n229 = Index Array(array=w336, index=w335) -> (element=w332:cluster{"Name":string, "Include":bool})
          n230 = Bundle By Name(cluster=w332, "Name"=w328) -> (w331:cluster{"Name":string, "Include":bool})
          n231 = Bundle By Name(cluster=w333, "Name"=w328, "Mean % Err"=w329, "% u'/U"=w329) -> (w330:T27)
        }
        n232 = Build Array (concatenate)("Nothing", w320) -> (w323:string[])
        n233 = local write "Block average display control"(w319) -> ()
        n234 = global write "Meas_global.vi" "Analysis type array"(w326) -> ()
        n235 = global write "Meas_global.vi" "Analysis Info cluster"(w324) -> ()
        n236 = global write "Meas_global.vi" "Velocity Cluster Array"(w318) -> ()
        n237 = property on="Plot 1" class="Ring (strict)"("Strings []"=w323) -> ()  [unwired: 2 in, 2 out]
        n238 = property on="Plot 1" class="Ring (strict)"("Strings []"=w323) -> ()  [unwired: 2 in, 2 out]
        n239 = property on="Plot 2" class="Ring (strict)"("Strings []"=w323) -> ()  [unwired: 2 in, 2 out]
        n240 = property on="Plot 2" class="Ring (strict)"("Strings []"=w323) -> ()  [unwired: 2 in, 2 out]
      }
      frame #11 {
        n241 = global read "Meas_global.vi" "Analysis Info cluster"() -> (w350:T20[])
        n242 = for {
          tunnel: w350 -> [w354] mode=indexing
          tunnel: [w353] -> w349 mode=indexing
          tunnel: [w352] -> w340
          i -> [w352]
          n243 = Unbundle By Name(w354) -> ("Inst name"=w353:string)
        }
        n244 = Greater Than 0?(x=w340) -> (x > 0?=w339:bool)
        n245 = Select(t="Correlate?", s=w339, f=T6."Cross correlation off" ("Correlate?")) -> (s? t:f=w341:T6)
        n246 = case shown="\"Correlate without activating panel\"" w341 {
          tunnel: w349 -> [_ w359 w361]
          tunnel: [w356 w358 w360] -> w338
          frame "Cross correlation off" {
            n247 = Initialize Array(0) -> (w356:i32[][])  [unwired: 2 out]
          }
          frame "Show correlation panel" {
            w357 = FALSE  # OK
            n248 = call "Correlation_Display.vi"("Inst names"=w359, "OK"=w357) -> ("correlation array"=w358:i32[][])  [unwired: 2 in, 2 out]
          }
          frame "Correlate without activating panel" {
            n249 = call "Correlation_Display.vi"("Inst names"=w361, "OK"=TRUE) -> ("correlation array"=w360:i32[][])  [unwired: 2 in, 2 out]
          }
        }
        n250 = global read "Meas_global.vi" "Position"() -> (w348:T7)
        n251 = local write "Position"(w348) -> ()
        n252 = global write "Meas_global.vi" "correlate"(w338) -> ()
        n253 = Array Size(array=w338) -> (size(s)=w347:i32[])
        n254 = Index Array(array=w347, index=0) -> (element=w345:i32)
        n255 = Equal To 0?(x=w345) -> (x = 0?=w344:bool)
        n256 = case shown="True" w344 {
          frame False {
          }
          frame True {
            n257 = local write "Correlate?"(T6."Cross correlation off" ("Correlate?")) -> ()
          }
        }
      }
      frame #12 {
        n258 = stacked-sequence {
          seq-local: [w369 _] -> [_ w391]
          tunnel: w363 -> [w368 _]
          frame #0 {
            n259 = call "LDA+_An_Analysis_mode.vi"("Second Graph"="Second Graph", "First Graph"="First Graph") -> ("Second Graph out"=w364:T3, "First Graph out"=w366:T3)  [unwired: 6 out]
            n260 = case shown="False" w368 {
              tunnel: [w379 w390] -> w367
              tunnel: w366 -> [w378 w390]
              tunnel: [w377 w389] -> w365
              tunnel: w364 -> [w376 w389]
              frame False {
                w374 = Graph_Type."Show no graph" ("Plot Type")
                n261 = Unbundle By Name(w378) -> ("Save graph"=w380:u16)
                n262 = Unbundle By Name(w376) -> ("Save graph"=w375:u16)
                n263 = case shown="0, Default" w380 {
                  tunnel: [w386 w388] -> w379
                  tunnel: w378 -> [w387 w388]
                  tunnel: w374 -> [w385 _]
                  frame 0, Default {
                    n264 = Bundle By Name(cluster=w387, "Plot Type"=w385) -> (w386:T3)
                  }
                  frame 1 {
                  }
                }
                n265 = case shown="0, Default" w375 {
                  tunnel: [w382 w384] -> w377
                  tunnel: w376 -> [w383 w384]
                  tunnel: w374 -> [w381 _]
                  frame 0, Default {
                    n266 = Bundle By Name(cluster=w383, "Plot Type"=w381) -> (w382:T3)
                  }
                  frame 1 {
                  }
                }
              }
              frame True {
              }
            }
            n267 = local write "Second Graph"(w365) -> ()
            n268 = local write "First Graph"(w367) -> ()
            n269 = global write "Meas_global.vi" "Second Graph"(w365) -> ()
            n270 = global write "Meas_global.vi" "First Graph"(w367) -> ()
            n271 = Unbundle By Name(w365) -> ("Plot Type"=w373:T2)
            n272 = Unbundle By Name(w367) -> ("Plot Type"=w372:T2)
            n273 = Build Array(w372, w373) -> (w369:T2[])
          }
          frame #1 {
            n274 = global read "Meas_global.vi" "Insts for plotting"() -> (w392:u16[][])
            n275 = for {
              tunnel: w392 -> [w394] mode=indexing
              tunnel: w391 -> [w393] mode=indexing
              i -> [w395]
              n276 = stacked-sequence {
                seq-local: [w398 _] -> [_ w408]
                seq-local: [w399 _] -> [_ w407]
                tunnel: w395 -> [_ w411]
                tunnel: w394 -> [w397 _]
                tunnel: w393 -> [_ w403]
                frame #0 {
                  n277 = property on="Plot 1" class="Ring (strict)"() -> ("Strings []"=w396:string[])  [unwired: 2 in, 2 out]
                  n278 = Array To Cluster(array=w397) -> (cluster=w402:T30)
                  n279 = Unbundle(w402) -> ("Insts for plotting[0]"=w401:u16, "Insts for plotting[1]"=w400:u16)
                  n280 = Index Array(array=w396, index=w401) -> (element=w398:string)
                  n281 = Index Array(array=w396, index=w400) -> (element=w399:string)
                }
                frame #1 {
                  n282 = case shown="\"Auto-Corr\"" w403 {
                    tunnel: [u8 0 u8 0 u8 0 u8 0 u8 0 u8 1 u8 0] -> w415
                    tunnel: [u8 0 u8 0 u8 0 u8 0 u8 1 u8 1 u8 0] -> w414
                    tunnel: [u8 0 u8 0 u8 0 u8 0 u8 1 u8 1 u8 0] -> w413
                    tunnel: [u8 0 u8 0 u8 0 u8 0 u8 1 u8 0 u8 0] -> w412
                    tunnel: [FALSE TRUE TRUE TRUE TRUE TRUE TRUE] -> w406
                    tunnel: [u8 0 u8 0 u8 0 u8 2 u8 0 u8 0 u8 2] -> w405
                    tunnel: [u8 0 u8 4 u8 1 u8 2 u8 0 u8 0 u8 1] -> w404
                    frame "Show no graph" {
                    }
                    frame "Voltage trace" {
                    }
                    frame "Velocity trace" {
                    }
                    frame "Vel histogram" {
                    }
                    frame "Spectrum" {
                    }
                    frame "f.E(f) v Log f" {
                    }
                    frame "Auto-Corr" {
                    }
                  }
                  n283 = case shown="0, Default" w411 {
                    tunnel: w406 -> [w426 w437]
                    tunnel: w415 -> [w425 w436]
                    tunnel: w414 -> [w424 w435]
                    tunnel: w413 -> [w423 w434]
                    tunnel: w412 -> [w422 w433]
                    tunnel: u32 0 -> [w421 w432]
                    tunnel: u32 1 -> [w420 w430]
                    tunnel: w408 -> [w419 w431]
                    tunnel: w407 -> [w418 w429]
                    tunnel: w405 -> [w417 w428]
                    tunnel: w404 -> [w416 w427]
                    frame 0, Default {
                      n284 = property on="First plot" class="WFGraph (strict)"("Visible"=w426, "X Scale.Format & Precision:Format"=w425, "X Scale.Mapping Mode"=w424, "Y Scale.Format & Precision:Format"=w423, "Y Scale.Mapping Mode"=w422, "Active Plot"=w421, "Plot.Plot Name"=w419, "Active Plot"=w420, "Plot.Plot Name"=w418, "X Scale.Format & Precision:Precision"=w417, "Y Scale.Format & Precision:Precision"=w416) -> ()  [unwired: 2 in, 2 out]
                    }
                    frame 1 {
                      n285 = property on="2nd plot" class="WFGraph (strict)"("Visible"=w437, "X Scale.Format & Precision:Format"=w436, "X Scale.Mapping Mode"=w435, "Y Scale.Format & Precision:Format"=w434, "Y Scale.Mapping Mode"=w433, "Active Plot"=w432, "Plot.Plot Name"=w431, "Active Plot"=w430, "Plot.Plot Name"=w429, "X Scale.Format & Precision:Precision"=w428, "Y Scale.Format & Precision:Precision"=w427) -> ()  [unwired: 2 in, 2 out]
                    }
                  }
                }
              }
            }
          }
        }
      }
      frame #13 {
        n286 = local read "Second Graph"() -> (w498:T3)
        n287 = local read "First Graph"() -> (w497:T3)
        n288 = Unbundle By Name(w497) -> ("Plot 1"=w490:u16, "Plot 2"=w491:u16)
        n289 = Unbundle By Name(w498) -> ("Plot 1"=w492:u16, "Plot 2"=w493:u16)
        n290 = Build Array(w490, w491) -> (w494:u16[])
        n291 = Build Array(w492, w493) -> (w495:u16[])
        n292 = global read "Meas_global.vi" "Analysis Info cluster"() -> (w499:T20[])
        n293 = Decrement(x=w494) -> (x-1=w488:u16[])
        n294 = Decrement(x=w495) -> (x-1=w496:u16[])
        n295 = for {
          tunnel: w499 -> [w507]
          tunnel: w488 -> [w506] mode=indexing
          shift-right: [w500] -> _
          shift-left: u32 0 -> [w502]
          i -> [w501]
          n296 = Index Array(array=w507, index=w506) -> (element=w508:T20)
          n297 = Unbundle By Name(w508) -> ("Colour"=w503:u32)
          n298 = Equal?(x=w503, y=w502) -> (x = y?=w505:bool)
          n299 = Select(t=u32 13434624, s=w505, f=w503) -> (s? t:f=w500:u32)
          n300 = property on="First plot" class="WFGraph (strict)"("Active Plot"=w501, "Plot.Plot Color"=w500, "Plot.Fill/Point Color"=w500) -> ()  [unwired: 2 in, 2 out]
        }
        n301 = for {
          tunnel: w499 -> [w516]
          tunnel: w496 -> [w515] mode=indexing
          shift-right: [w511] -> _
          shift-left: u32 0 -> [w509]
          i -> [w514]
          n302 = Index Array(array=w516, index=w515) -> (element=w517:T20)
          n303 = Unbundle By Name(w517) -> ("Colour"=w510:u32)
          n304 = Equal?(x=w510, y=w509) -> (x = y?=w513:bool)
          n305 = Select(t=u32 13434624, s=w513, f=w510) -> (s? t:f=w511:u32)
          n306 = property on="2nd plot" class="WFGraph (strict)"("Active Plot"=w514, "Plot.Plot Color"=w511, "Plot.Fill/Point Color"=w511) -> ()  [unwired: 2 in, 2 out]
        }
      }
      frame #14 {
        n307 = global read "DataTranslation_global.vi" "Different Sampling Freq per block"() -> (w518:bool)
        n308 = global read "Meas_global.vi" "Remote control"() -> (w527:bool)
        n309 = global read "Meas_global.vi" "Post Process"() -> (w530:T5)
        n310 = global read "Meas_global.vi" "PWA Data"() -> (w519:T31)
        n311 = case shown="\"One Ch PWA\"" w519 {
          tunnel: [w531 w536] -> w521
          frame "No PWA Data" {
            n312 = local read "Desired Sampling freq (Hz)"() -> (w533:dbl)
            n313 = local read "No of samples"() -> (w532:i32)
            n314 = Divide(x=w532, y=w533) -> (x/y=w531:dbl)
          }
          frame "One Ch PWA" {
            n315 = local read "No of samples"() -> (w534:i32)
            n316 = global read "PWAtasksGLOBAL.vi" "PWA Freq. (Hz)"() -> (w535:dbl)
            n317 = global write "PWAtasksGLOBAL.vi" "PWA No. of Samples"(w534) -> ()
            n318 = Divide(x=w534, y=w535) -> (x/y=w536:dbl)
          }
        }
        n319 = global read "Meas_global.vi" "Averaging time (min)"() -> (w525:dbl)
        n320 = Equal?(x=Setup."Run Program" ("setup"), y=w524) -> (x = y?=w522:bool)
        n321 = Equal?(x=Post_Process."Take New Data" ("Post Process"), y=w530) -> (x = y?=w526:bool)
        n322 = Compound Arithmetic op=AND(invert w518, w526, invert w520, invert w527, w522) -> (w528:bool)
        n323 = case shown="True" w528 {
          tunnel: w525 -> [_ w547]
          tunnel: w521 -> [_ w546]
          tunnel: w519 -> [_ w542]
          frame False {
          }
          frame True {
            n324 = global read "Meas_global.vi" "Board type"() -> (w544:T13)
            n325 = Equal?(x=w544, y=Board_Types."Simulate" ("Board type")) -> (x = y?=w538:bool)
            n326 = global read "Meas_global.vi" "LDA data"() -> (w540:enum16{"No LDA data", "Take LDA data"})
            n327 = Equal?(x=enum16{"No LDA data", "Take LDA data"}."Take LDA data" ("LDA data"), y=w540) -> (x = y?=w539:bool)
            n328 = Compound Arithmetic op=AND(invert w539, w538) -> (w537:bool)
            n329 = case shown="False" w537 {
              tunnel: w547 -> [w557 _]
              tunnel: w546 -> [w551 _]
              tunnel: [w550 1 ("No of Blocks")] -> w543
              tunnel: w542 -> [w549 _]
              tunnel: w539 -> [w548 _]
              frame False {
                n330 = Multiply(x=w557, y=60.0) -> (x*y=w555:dbl)
                n331 = Divide(x=w555, y=w551) -> (x/y=w554:dbl)
                n332 = Round Toward +Infinity(x=w554) -> (ceil(x): smallest int >= x=w553:dbl)
                n333 = To Long Integer(number=w553) -> (32bit integer=w552:i32)
                n334 = case shown="\"No PWA Data\"" w549 {
                  tunnel: w548 -> [w561 _]
                  tunnel: w552 -> [w559 w562]
                  tunnel: [w558 w562] -> w550
                  frame "No PWA Data" {
                    n335 = Select(t=99999 ("No of Blocks"), s=w561, f=w559) -> (s? t:f=w558:i32)
                  }
                  frame "One Ch PWA" {
                  }
                }
              }
              frame True {
              }
            }
            n336 = global write "Meas_global.vi" "Requested No of blocks"(w543) -> ()
            n337 = local write "No of Blocks"(w543) -> ()
          }
        }
      }
      frame #15 {
        n338 = case shown="\"Run Program\"" w564 {
          frame "Run Program" {
            n339 = call "Read_calibration_files.vi"() -> ()  [unwired: 1 out]
            n340 = global write "Meas_global.vi" "Repeat Measurement?"(FALSE ("Repeat Measurement?")) -> ()
          }
          frame "Show Setup", Default {
          }
        }
      }
      frame #16 {
        n341 = global read "Meas_global.vi" "Raw data option"() -> (w569:enum16{"Save raw data", "Raw data not saved"})
        n342 = Get Date/Time In Seconds() -> (seconds since 1Jan1904=w570:timestamp)
        n343 = To Double Precision Float(number=w570) -> (double precision float=w567:dbl)
        n344 = global read "Meas_global.vi" "Post Process"() -> (w568:T5)
        n345 = case shown="\"Setup Front Panel\"" w571 {
          tunnel: w569 -> [w574 _ _ _]
          tunnel: w568 -> [w573 _ w606 w615]
          frame "Run Program" {
            n346 = case shown="\"Take New Data\"" w573 {
              tunnel: w574 -> [w575 _]
              frame "Take New Data" {
                n347 = case shown="\"Raw data not saved\"" w575 {
                  frame "Save raw data" {
                  }
                  frame "Raw data not saved" {
                    w583 = FALSE  # Lock File
                    w580 = FALSE  # advisory dialog? (display:T)
                    w579 = FALSE  # append to file? (new file:F)
                    n348 = global read "Meas_global.vi" "Remote control"() -> (w581:bool)
                    n349 = call "Create_setup_string.vi"() -> ("Setup String"=w584:string)  [unwired: 1 out]
                    n350 = case shown="False" w581 {
                      tunnel: ["Current_Setup.xls" ("Setup filename") w586] -> w576
                      frame False {
                      }
                      frame True {
                        n351 = local read "Setup filename"() -> (w586:string)
                      }
                    }
                    n352 = call "Add_length_to_string.vi"("String in"=w584) -> ("String out"=w582:string)
                    n353 = call "Setup_Filepath.vi"("Setup File Type"=Setup_Filetype."Measurement Setups", "Filename in"=w576) -> ("Filename Out"=w577:path)  [unwired: 1 out]
                    n354 = call "Write_Characters_To_File.vi"("file path (dialog if empty)"=w577, "advisory dialog? (display:T)"=w580, "character string"=w582, "append to file? (new file:F)"=w579, "Lock File"=w583) -> ()  [unwired: 4 out]
                  }
                }
              }
              frame "Post Process Raw Data File" {
              }
            }
          }
          frame "Save Current Setup" {
            n355 = stacked-sequence {
              seq-local: [w589 _] -> [_ w592]
              seq-local: [w588 _] -> [_ w591]
              frame #0 {
                w590 = FALSE  # Save New File?
                n356 = call "Save_current_setup.vi"("Save New File?"=w590, "Setup File Type"=Setup_Filetype."Measurement Setups") -> ("Cancelled?"=w588:bool, "Saved filepath"=w589:path)  [unwired: 2 out]
              }
              frame #1 {
                n357 = case shown="False" w591 {
                  tunnel: w592 -> [w598 _]
                  frame False {
                    w595 = "Initial Probe positions" ("File Label")
                    w603 = FALSE  # append to file? (new file:F)
                    w604 = FALSE  # advisory dialog? (display:T)
                    w605 = FALSE  # Lock File
                    n358 = call "Input_Instrument_Positions.vi"("Filepath to Save"=w598) -> ("Output string"=w597:string)  [unwired: 1 out]
                    n359 = call "Create_setup_string.vi"() -> ("Setup String"=w596:string)  [unwired: 1 out]
                    n360 = call "Get_string_subset.vi"("String to split"=w597, "File Label"=w595) -> ("Output string"=w594:string)  [unwired: 2 in, 1 out]
                    n361 = call "Replace_data_in_Label_str.vi"("New data string"=w594, "Input string"=w596, "Variable name"=w595) -> ("Appended string"=w593:string)
                    n362 = call "Replace_data_in_setup_string.vi"("New data string"="", "Input string"=w593, "Variable name"="Comments") -> ("Appended string"=w599:string)
                    n363 = call "Add_length_to_string.vi"("String in"=w599) -> ("String out"=w602:string)
                    n364 = call "Write_Characters_To_File.vi"("file path (dialog if empty)"=w598, "advisory dialog? (display:T)"=w604, "character string"=w602, "append to file? (new file:F)"=w603, "Lock File"=w605) -> ()  [unwired: 4 out]
                  }
                  frame True {
                  }
                }
              }
            }
          }
          frame "Show Setup" {
            n365 = case shown="\"Take New Data\"" w606 {
              frame "Take New Data" {
                w611 = FALSE  # append to file? (new file:F)
                w612 = FALSE  # advisory dialog? (display:T)
                w613 = FALSE  # Lock File
                n366 = call "Create_setup_string.vi"() -> ("Setup String"=w614:string)  [unwired: 1 out]
                n367 = call "Add_length_to_string.vi"("String in"=w614) -> ("String out"=w610:string)
                n368 = call "Setup_Filepath.vi"("Setup File Type"=Setup_Filetype."Measurement Setups", "Filename in"="Current_Setup.xls" ("Setup filename")) -> ("Filename Out"=w608:path)  [unwired: 1 out]
                n369 = call "Write_Characters_To_File.vi"("file path (dialog if empty)"=w608, "advisory dialog? (display:T)"=w612, "character string"=w610, "append to file? (new file:F)"=w611, "Lock File"=w613) -> ()  [unwired: 4 out]
              }
              frame "Post Process Raw Data File" {
              }
            }
          }
          frame "Setup Front Panel" {
            n370 = case shown="\"Take New Data\"" w615 {
              frame "Take New Data" {
                w620 = FALSE  # append to file? (new file:F)
                w621 = FALSE  # advisory dialog? (display:T)
                w622 = FALSE  # Lock File
                n371 = call "Create_setup_string.vi"() -> ("Setup String"=w623:string)  [unwired: 1 out]
                n372 = call "Add_length_to_string.vi"("String in"=w623) -> ("String out"=w619:string)
                n373 = call "Setup_Filepath.vi"("Setup File Type"=Setup_Filetype."Measurement Setups", "Filename in"="Current_Setup.xls" ("Setup filename")) -> ("Filename Out"=w617:path)  [unwired: 1 out]
                n374 = call "Write_Characters_To_File.vi"("file path (dialog if empty)"=w617, "advisory dialog? (display:T)"=w621, "character string"=w619, "append to file? (new file:F)"=w620, "Lock File"=w622) -> ()  [unwired: 4 out]
              }
              frame "Post Process Raw Data File" {
              }
            }
          }
        }
        n375 = call "Program_Active.vi"() -> ()  [unwired: 1 in]
        n376 = global write "Meas_global.vi" "Actual Measurement time (min)"(0.0 ("Max Measurement time (min)")) -> ()
        n377 = global write "Meas_global.vi" "Current Block No"(0 ("Current Block No")) -> ()
      }
      frame #17 {
        n378 = case shown="\"Run Program\"" w627 {
          tunnel: w624 -> [w629 _]
          tunnel: w626 -> [_ w816]
          tunnel: w625 -> [w628 _]
          frame "Run Program" {
            # "PWA"
            # "LDA"
            # "An"
            n379 = stacked-sequence {
              seq-local: [w637 _] -> [_ w659]
              seq-local: [w636 _] -> [_ w658]
              seq-local: [w635 _] -> [_ w657]
              seq-local: [w633 _] -> [_ w656]
              seq-local: [w631 _] -> [_ w653]
              seq-local: [w630 _] -> [_ w652]
              tunnel: w629 -> [_ w655]
              tunnel: w628 -> [_ w654]
              frame #0 {
                n380 = global read "Trav_pos_global.vi" "Dummy Measurement?"() -> (w632:bool)
                n381 = case shown="False" w632 {
                  tunnel: [w644 u16[][] [] ("LDA Binary output")] -> w637
                  tunnel: [w643 w646] -> w636
                  tunnel: [w642 dbl[][] [] ("Voltage output")] -> w635
                  tunnel: [w641 TRUE ("EOF?")] -> w634
                  tunnel: [w640 T15 {"Started"=0.0, "Ended"=0.0, "Analogue Frequency Hz"=1000.0} ("Block Timings")] -> w633
                  tunnel: [w639 w646] -> w631
                  tunnel: [w638 ""] -> w630
                  frame False {
                    n382 = call "Get_data.vi"() -> ("EOF? and Error status"=w641:bool, "Voltage output"=w642:dbl[][], "Analogue Binary"=w643:i16[][], "LDA Binary output"=w644:u16[][], "Block Timings"=w640:T15, "PWA Binary"=w639:i16[][], "Block Header"=w638:string)  [unwired: 5 out]
                  }
                  frame True {
                    w646 = i16[][] [] ("Analogue Binary")
                  }
                }
                n383 = case shown="True" w634 {
                  frame False {
                  }
                  frame True {
                    n384 = local write "No of Blocks"(1 ("No of Blocks")) -> ()
                  }
                }
              }
              frame #1 {
                n385 = while {
                  tunnel: w655 -> [w665]
                  shift-left: w656 -> [w666]
                  shift-right: [w667] -> _
                  shift-left: w657 -> [w671]
                  shift-right: [w674] -> _
                  shift-left: w658 -> [w672]
                  shift-right: [w675] -> _
                  shift-left: w659 -> [w673]
                  shift-right: [w676] -> _
                  tunnel: w654 -> [w664]
                  shift-right: [w663] -> _
                  shift-left: w653 -> [w662]
                  shift-right: [w661] -> _
                  shift-left: w652 -> [w660]
                  i -> [w668]
                  stop <- w677 continue-if-true
                  n386 = Increment(x=w668) -> (x+1=w678:i32)
                  n387 = stacked-sequence {
                    seq-local: [_ _ _ _ _ "Block average display control" _ _ _ _] -> [_ _ _ _ _ _ w773 _ _ _]
                    seq-local: [_ _ _ _ _ _ w770 _ _ _] -> [_ _ _ _ _ _ _ w784 _ _]
                    seq-local: [w714 _ _ _ _ _ _ _ _ _] -> [_ w720 _ _ w756 _ _ _ _ w814]
                    seq-local: [_ _ w725 _ _ _ _ _ _ _] -> [_ _ _ _ w754 _ _ _ _ _]
                    seq-local: [_ _ _ w746 _ _ _ _ _ _] -> [_ _ _ _ w755 _ _ _ _ _]
                    tunnel: w678 -> [w713 _ _ _ w758 w766 _ _ _ _]
                    tunnel: [_ _ _ _ _ _ _ _ _ w814] -> w677
                    tunnel: w668 -> [_ _ _ _ _ _ _ _ _ _]
                    tunnel: w673 -> [_ _ _ w744 _ _ _ _ _ _]
                    tunnel: w672 -> [_ _ _ w743 _ _ _ _ _ _]
                    tunnel: w671 -> [_ _ _ w750 _ _ _ _ _ _]
                    tunnel: "stop" -> [w716 _ _ _ _ _ _ _ _ _]
                    tunnel: "No of Blocks" -> [w715 _ _ _ _ _ _ _ _ _]
                    tunnel: w666 -> [_ _ _ w748 _ _ _ _ _ _]
                    tunnel: w665 -> [_ _ w724 w745 _ _ _ _ _ _]
                    tunnel: w664 -> [_ _ w726 _ _ _ _ _ _ _]
                    tunnel: w662 -> [_ _ _ w742 _ _ _ _ _ _]
                    tunnel: w660 -> [w712 _ _ _ _ _ _ _ _ _]
                    frame #0 {
                      n388 = global write "Plug_in_data_global.vi" "Block Header"(w712) -> ()
                      n389 = Less Or Equal?(x=w715, y=w713) -> (x <= y?=w718:bool)
                      n390 = Or(x=w716, y=w718) -> (x .or. y?=w717:bool)
                      n391 = global write "Meas_global.vi" "Current Block No"(w713) -> ()
                      n392 = Not(x=w717) -> (.not. x?=w714:bool)
                    }
                    frame #1 {
                      n393 = call "Program_Active.vi"() -> ()  [unwired: 1 in]
                      n394 = call "Text_without_format.vi"("Input string"="Comments") -> ("Output string"=w721:string)
                      n395 = global write "Meas_global.vi" "Position"("Position") -> ()
                      n396 = local write "Comments"(w721) -> ()
                      n397 = global write "Meas_global.vi" "Comments"(w721) -> ()
                      n398 = Not(x=w720) -> (.not. x?=w719:bool)
                      n399 = global write "Meas_global.vi" "Processing last block?"(w719) -> ()
                      n400 = global write "PWAtasksGLOBAL.vi" "STOP"(w719) -> ()
                    }
                    frame #2 {
                      n401 = case shown="False" w724 {
                        tunnel: w726 -> [w738 _]
                        tunnel: [w727 FALSE] -> w725
                        frame False {
                          w735 = 1.5  # To allow for overhead
                          n402 = Get Date/Time In Seconds() -> (seconds since 1Jan1904=w740:timestamp)
                          n403 = global read "Meas_global.vi" "Averaging time (min)"() -> (w734:dbl)
                          n404 = To Double Precision Float(number=w740) -> (double precision float=w739:dbl)
                          n405 = Subtract(x=w739, y=w738) -> (x-y=w737:dbl)
                          n406 = global read "Meas_global.vi" "LDA data"() -> (w731:enum16{"No LDA data", "Take LDA data"})
                          n407 = Divide(x=w737, y=60.0 ("To convert to minutes")) -> (x/y=w733:dbl)
                          n408 = Equal?(x=enum16{"No LDA data", "Take LDA data"}."Take LDA data" ("LDA data"), y=w731) -> (x = y?=w728:bool)
                          n409 = Multiply(x=w735, y=w734) -> (x*y=w732:dbl)
                          n410 = Greater?(x=w733, y=w732) -> (0:w729:bool)
                          n411 = And(x=w728, y=w729) -> (x .and. y?=w727:bool)
                        }
                        frame True {
                        }
                      }
                    }
                    frame #3 {
                      n412 = call "Process_data.vi"("PWA Binary"=w742, "Analogue Binary"=w743, "LDA Binary output"=w744, "Analogue volts"=w750, "Measurement top level?"=w745, "Block Timings"=w748) -> ("Vel stat display"=→"Statistics":string[][], "First Plot data"=→"First plot":cluster{"Xo":dbl, "Delta X":dbl, dbl[]}[], "Second Plot data"=→"2nd plot":cluster{"Xo":dbl, "Delta X":dbl, dbl[]}[], "Max Measurement time up"=w746:bool)
                    }
                    frame #4 {
                      n413 = global read "Meas_global.vi" "stop"() -> (w753:bool)
                      n414 = Compound Arithmetic op=OR(w753, w754, w755) -> (w752:bool)
                      n415 = And(x=w756, y=w752) -> (x .and. y?=w757:bool)
                      n416 = case shown="True" w757 {
                        tunnel: w758 -> [_ w759]
                        frame False {
                        }
                        frame True {
                          n417 = Increment(x=w759) -> (x+1=w760:i32)
                          n418 = local write "No of Blocks"(w760) -> ()
                        }
                      }
                    }
                    frame #5 {
                      n419 = global read "Meas_global.vi" "Actual Measurement time (min)"() -> (→"Measurement time (min)":dbl)
                      n420 = global read "Meas_global.vi" "Actual Sampling rate (Hz)"() -> (→"Actual Sampling freq":dbl)
                      n421 = call "Display_blocks.vi"("Block No"=w766, "Block average display"="Block average display control") -> ("u^4"=→"u^4":dbl[][], "u^3"=→"u^3":dbl[][], "uv"=→"uv":dbl[][], "u^2"=→"u^2" →"Array u^2":dbl[][], "U"=→"U" →"Array U":dbl[][])  [unwired: 4 out]
                    }
                    frame #6 {
                      n422 = global read "Meas_global.vi" "Analysis Info cluster"() -> (w772:T20[])
                      n423 = for {
                        tunnel: w773 -> [w778] mode=indexing
                        shift-right: [w774] -> w770
                        shift-left: u32[] [] -> [w775]
                        tunnel: w772 -> [w777] mode=indexing
                        n424 = Unbundle By Name(w778) -> ("Include"=w776:bool)
                        n425 = case shown="True" w776 {
                          tunnel: w777 -> [_ w783]
                          tunnel: w775 -> [w779 w781]
                          tunnel: [w779 w780] -> w774
                          frame False {
                          }
                          frame True {
                            n426 = Unbundle By Name(w783) -> ("Colour"=w782:u32)
                            n427 = Build Array (concatenate)(w781, w782) -> (w780:u32[])
                          }
                        }
                      }
                    }
                    frame #7 {
                      n428 = for {
                        tunnel: w784 -> [w785] mode=indexing
                        i -> [w786]
                        n429 = property on="U" class="WFGraph (strict)"("Active Plot"=w786, "Plot.Plot Color"=w785, "Plot.Fill/Point Color"=w785) -> ()  [unwired: 2 in, 2 out]
                        n430 = property on="u^3" class="WFGraph (strict)"("Active Plot"=w786, "Plot.Plot Color"=w785, "Plot.Fill/Point Color"=w785) -> ()  [unwired: 2 in, 2 out]
                        n431 = property on="u^4" class="WFGraph (strict)"("Active Plot"=w786, "Plot.Plot Color"=w785, "Plot.Fill/Point Color"=w785) -> ()  [unwired: 2 in, 2 out]
                        n432 = property on="u^2" class="WFGraph (strict)"("Active Plot"=w786, "Plot.Plot Color"=w785, "Plot.Fill/Point Color"=w785) -> ()  [unwired: 2 in, 2 out]
                      }
                    }
                    frame #8 {
                      n433 = case shown="True" "Pause" {
                        frame False {
                        }
                        frame True {
                          n434 = global read "Meas_global.vi" "Post Process"() -> (w788:T5)
                          n435 = case shown="\"Take New Data\"" w788 {
                            frame "Take New Data" {
                              n436 = call "Program_Active_Client.vi"("Mode"=enum16{"Program Active", "Traverse Level State"}."Program Active", "Time till next contact (Sec)"=12000.0, "Traverse level State"=Traverse_Level_State."Running") -> ()  [unwired: 3 out]
                              n437 = while {
                                i -> [w795]
                                stop <- w796 continue-if-true
                                n438 = Quotient & Remainder(x=w795, y=10) -> (x-y*floor(x/y)=w793:i32)  [unwired: 1 out]
                                n439 = Equal To 0?(x=w793) -> (x = 0?=w792:bool)
                                n440 = stacked-sequence {
                                seq-local: [_ w798 _ _] -> [_ _ w800 _]
                                tunnel: [_ w798 _ _] -> w796
                                tunnel: w792 -> [_ _ _ w802]
                                frame #0 {
                                "Pause message" <- "Measurement Program Paused!!!!" ("Pause message")
                                }
                                frame #1 {
                                n441 = global write "Trav_pos_global.vi" "Paused During Row?"(TRUE ("Paused During Row?")) -> ()
                                n442 = local read "Pause"() -> (w798:bool)
                                }
                                frame #2 {
                                n443 = property on="Pause message" class="Str"("Blinking"=w800, "Visible"=w800) -> ()  [unwired: 2 in, 2 out]
                                n444 = Wait Until Next ms Multiple(millisecond multiple=u32 1000) -> ()  [unwired: 1 out]
                                }
                                frame #3 {
                                n445 = case shown="False" w802 {
                                frame False {
                                }
                                frame True {
                                n446 = Current VI's Path() -> (path=w803:path)
                                n447 = call "Bring_to_front.vi"("path"=w803) -> ()
                                }
                                }
                                }
                                }
                              }
                            }
                            frame "Post Process Raw Data File" {
                              n448 = stacked-sequence {
                                seq-local: [_ w806 _ _] -> [_ _ _ w813]
                                frame #0 {
                                n449 = property on="PP next block" class="Bool (strict)"("Visible"=TRUE) -> ()  [unwired: 2 in, 2 out]
                                n450 = local write "PP next block"(FALSE ("PP next block")) -> ()
                                }
                                frame #1 {
                                n451 = while {
                                tunnel: [w810] -> w806
                                stop <- w807 stop-if-true
                                n452 = local read "stop"() -> (w810:bool)
                                n453 = local read "Pause"() -> (w808:bool)
                                n454 = Compound Arithmetic op=OR(w810, "PP next block", invert w808) -> (w807:bool)
                                n455 = case shown="False" w807 {
                                frame False {
                                n456 = Wait (ms)(milliseconds to wait=u32 200) -> ()  [unwired: 1 out]
                                }
                                frame True {
                                }
                                }
                                }
                                }
                                frame #2 {
                                n457 = property on="PP next block" class="Bool (strict)"("Visible"=FALSE) -> ()  [unwired: 2 in, 2 out]
                                }
                                frame #3 {
                                n458 = Stop(stop? (T)=w813) -> ()
                                }
                              }
                            }
                          }
                        }
                      }
                    }
                    frame #9 {
                      n459 = global read "Meas_global.vi" "Diagnostic info"() -> (→"BSA Diagnostic info":string[][])
                    }
                  }
                  n460 = stacked-sequence {
                    seq-local: [w680 _ _] -> [_ w690 _]
                    seq-local: [_ w689 _] -> [_ _ w710]
                    tunnel: [_ w693 _] -> w676
                    tunnel: [_ w692 _] -> w675
                    tunnel: [_ w691 _] -> w674
                    tunnel: "No of Blocks" -> [w685 _ _]
                    tunnel: "stop" -> [w683 _ _]
                    tunnel: w668 -> [w681 _ w709]
                    tunnel: [_ w688 _] -> w667
                    tunnel: [_ w687 _] -> w663
                    tunnel: [_ w686 _] -> w661
                    frame #0 {
                      n461 = Increment(x=w681) -> (x+1=w679:i32)
                      "Current Block No" <- w679
                      n462 = Less Or Equal?(x=w685, y=w679) -> (x <= y?=w684:bool)
                      n463 = Or(x=w684, y=w683) -> (x .or. y?=w682:bool)
                      n464 = Not(x=w682) -> (.not. x?=w680:bool)
                      n465 = global write "Meas_global.vi" "Current Block No"(w679) -> ()
                    }
                    frame #1 {
                      n466 = case shown="True" w690 {
                        tunnel: [u16[][] [] ("LDA Binary output") w706] -> w693
                        tunnel: [w695 w705] -> w692
                        tunnel: [dbl[][] [] ("Voltage output") w704] -> w691
                        tunnel: [FALSE ("EOF?") w703] -> w689
                        tunnel: [T15 {"Started"=0.0, "Ended"=0.0, "Analogue Frequency Hz"=200.0} ("Block Timings") w702] -> w688
                        tunnel: [w695 w701] -> w687
                        tunnel: ["" w700] -> w686
                        frame False {
                          w695 = i16[][] [] ("Analogue Binary")
                        }
                        frame True {
                          n467 = call "Get_data.vi"() -> ("EOF? and Error status"=w703:bool, "Voltage output"=w704:dbl[][], "Analogue Binary"=w705:i16[][], "LDA Binary output"=w706:u16[][], "Block Timings"=w702:T15, "PWA Binary"=w701:i16[][], "Block Header"=w700:string)  [unwired: 5 out]
                        }
                      }
                    }
                    frame #2 {
                      n468 = Increment(x=w709) -> (x+1=w707:i32)
                      n469 = Increment(x=w707) -> (x+1=w708:i32)
                      n470 = case shown="True" w710 {
                        tunnel: w708 -> [_ w711]
                        frame False {
                        }
                        frame True {
                          n471 = local write "No of Blocks"(w711) -> ()
                        }
                      }
                    }
                  }
                }
              }
            }
          }
          frame "Setup Front Panel", Default {
            n472 = stacked-sequence {
              seq-local: [w817 _ _ _ _ _ _] -> [_ _ _ _ _ w891 _]
              seq-local: [_ w823 _ _ _ _ _] -> [_ _ _ _ _ w890 _]
              seq-local: [_ _ _ w854 _ _ _] -> [_ _ _ _ _ w889 _]
              seq-local: [_ _ _ _ w867 _ _] -> [_ _ _ _ _ w887 _]
              seq-local: [_ w822 _ _ _ _ _] -> [_ _ _ _ _ _ w904]
              seq-local: [_ _ w848 _ _ _ _] -> [_ _ _ _ _ w886 _]
              tunnel: w816 -> [_ w824 _ _ _ _ _]
              frame #0 {
                n473 = Build Array("Name", "Channel", "High limit", "Low limit") -> (w817:string[])
              }
              frame #1 {
                n474 = global read "Meas_global.vi" "LDA data"() -> (w822:enum16{"No LDA data", "Take LDA data"})
                n475 = case shown="\"Take LDA data\"" w822 {
                  tunnel: w824 -> [_ w835]
                  tunnel: [string[][] [] w832] -> w823
                  frame "No LDA data" {
                  }
                  frame "Take LDA data" {
                    n476 = case shown="\"2D\"" w835 {
                      tunnel: [string[] [] w841] -> w833
                      frame "1D" {
                      }
                      frame "2D" {
                        n477 = global read "LDA_meas_global_2.vi" "Max Vel BSA2"() -> (w840:dbl)
                        n478 = global read "LDA_meas_global_2.vi" "Min Vel BSA2"() -> (w839:dbl)
                        n479 = global read "LDA_meas_global_2.vi" "Vel Comp BSA2"() -> (w842:string)
                        n480 = Format Into String(format string="%.1f m/s" ("Format String"), w839) -> (resulting string=w847:string)  [unwired: 2 in, 1 out]
                        n481 = Format Into String(format string="%.1f m/s" ("Format String"), w840) -> (resulting string=w846:string)  [unwired: 2 in, 1 out]
                        n482 = Build Array("LDA", w842, w846, w847) -> (w841:string[])
                      }
                    }
                    n483 = global read "LDA_meas_global_1.vi" "Max Vel BSA1"() -> (w827:dbl)
                    n484 = global read "LDA_meas_global_1.vi" "Vel Comp BSA1"() -> (w836:string)
                    n485 = global read "LDA_meas_global_1.vi" "Min Vel BSA1"() -> (w826:dbl)
                    n486 = Format Into String(format string="%.1f m/s" ("Format String"), w826) -> (resulting string=w828:string)  [unwired: 2 in, 1 out]
                    n487 = Format Into String(format string="%.1f m/s" ("Format String"), w827) -> (resulting string=w829:string)  [unwired: 2 in, 1 out]
                    n488 = Build Array("LDA", w836, w829, w828) -> (w834:string[])
                    n489 = Build Array(w834, w833) -> (w832:string[][])
                  }
                }
              }
              frame #2 {
                n490 = global read "Meas_global.vi" "PWA Data"() -> (w849:T31)
                n491 = case shown="\"One Ch PWA\"" w849 {
                  tunnel: [string[][] [] w851] -> w848
                  frame "No PWA Data" {
                  }
                  frame "One Ch PWA" {
                    n492 = Build Array("PWA") -> (w852:string[])
                    n493 = Build Array(w852) -> (w851:string[][])
                  }
                }
              }
              frame #3 {
                n494 = global read "Meas_global.vi" "Ch & spans"() -> (w855:T26[])
                n495 = for {
                  tunnel: w855 -> [w866] mode=indexing
                  tunnel: [w862] -> w854 mode=indexing
                  n496 = Unbundle By Name(w866) -> ("Var name"=w865:string, "Ch No"=w864:i16, "high limit (10V)"=w859:sgl, "low limit (-10V)"=w858:sgl)
                  n497 = Format Into String(format string="%.1f Volts" ("Format String"), w859) -> (resulting string=w857:string)  [unwired: 2 in, 1 out]
                  n498 = Format Into String(format string="%.1f Volts" ("Format String"), w858) -> (resulting string=w856:string)  [unwired: 2 in, 1 out]
                  n499 = Number To Decimal String(number=w864) -> (decimal integer string=w863:string)  [unwired: 1 out]
                  n500 = Build Array(w865, w863, w857, w856) -> (w862:string[])
                }
              }
              frame #4 {
                n501 = global read "Meas_global.vi" "Analysis Info cluster"() -> (w875:T20[])
                n502 = for {
                  tunnel: w875 -> [w885] mode=indexing
                  tunnel: [w884] -> w873 mode=indexing
                  n503 = Unbundle By Name(w885) -> ("Inst name"=w884:string)
                }
                n504 = global read "Meas_global.vi" "correlate"() -> (w874:i32[][])
                n505 = for {
                  tunnel: w874 -> [w880] mode=indexing
                  tunnel: w873 -> [w879]
                  tunnel: "Correlating" -> [w878]
                  tunnel: [w876] -> w868 mode=indexing
                  n506 = for {
                    tunnel: w880 -> [w883] mode=indexing
                    tunnel: w879 -> [w882]
                    tunnel: [w881] -> w877 mode=indexing
                    n507 = Index Array(array=w882, index=w883) -> (element=w881:string)
                  }
                  n508 = Build Array (concatenate)(w878, w877) -> (w876:string[])
                }
                n509 = Initialize Array("", 5 ("Dimension Size")) -> (w869:string[])
                n510 = Build Array (concatenate)(w869, w868) -> (w867:string[][])
              }
              frame #5 {
                n511 = Build Array (concatenate)(w891, w890, w886, w889, w887) -> (w888:string[][])
                n512 = local write "Statistics"(w888) -> ()
              }
              frame #6 {
                n513 = global read "Meas_global.vi" "Board type"() -> (w902:T13)
                n514 = global read "Meas_global.vi" "Continuous time trace?"() -> (w903:bool)
                n515 = Equal?(x=w902, y=Board_Types."ADC488" ("Board type")) -> (x = y?=w900:bool)
                n516 = case shown="\"Take LDA data\"" w904 {
                  tunnel: w900 -> [_ w908]
                  tunnel: [string[] [] w907] -> w896
                  frame "No LDA data" {
                  }
                  frame "Take LDA data" {
                    n517 = global read "Meas_global.vi" "Synchronise with LDA"() -> (w913:bool)
                    n518 = global read "Meas_global.vi" "Ch & spans"() -> (w916:T26[])
                    n519 = global read "LDA_meas_global_1.vi" "Probe Configuration"() -> (w906:string)
                    n520 = Array Size(array=w916) -> (size(s)=w915:i32)
                    n521 = Greater Than 0?(x=w915) -> (x > 0?=w914:bool)
                    n522 = Compound Arithmetic op=AND(w913, w908, w914) -> (w912:bool)
                    n523 = Select(t="Synchronised with LDA", s=w912, f="") -> (s? t:f=w909:string)
                    n524 = Build Array(w906, w909) -> (w907:string[])
                  }
                }
                n525 = Compound Arithmetic op=AND(w900, w903) -> (w897:bool)
                n526 = Select(t="Continuous Time Trace", s=w897, f="") -> (s? t:f=w895:string)
                n527 = Build Array (concatenate)(w896, w895) -> (w894:string[])
                n528 = Build Array(w894) -> (w893:string[][])
                n529 = Transpose 2D Array(2D array=w893) -> (transposed array=w892:string[][])
                n530 = local write "BSA Diagnostic info"(w892) -> ()
              }
            }
          }
        }
      }
      frame #18 {
        n531 = local read "File"() -> (w934:T9)
        n532 = Equal?(x=Setup."Run Program" ("setup"), y=w935) -> (x = y?=w932:bool)
        n533 = Not Equal?(x=w934, y=Save_Data."Save No Data" ("File")) -> (x != y?=w933:bool)
        n534 = global read "Meas_global.vi" "Repeat Measurement?"() -> (w917:bool)
        n535 = Compound Arithmetic op=AND(invert w917, w932, w933) -> (w931:bool)
        n536 = Get Date/Time In Seconds() -> (seconds since 1Jan1904=w928:timestamp)
        n537 = To Double Precision Float(number=w928) -> (double precision float=w920:dbl)
        n538 = local read "Setup filename"() -> (w929:string)
        n539 = global read "Trav_pos_global.vi" "Meas Setup Number"() -> (w926:i32)
        n540 = global read "Meas_global.vi" "Board type"() -> (w924:T13)
        n541 = Greater Than 0?(x=w926) -> (x > 0?=w922:bool)
        n542 = Equal?(x=w924, y=Board_Types."Simulate" ("Board type")) -> (x = y?=w923:bool)
        n543 = And(x=w922, y=w923) -> (x .and. y?=w921:bool)
        n544 = case shown="True" w921 {
          tunnel: w920 -> [_ w939]
          tunnel: [w936 w937] -> w919
          tunnel: w918 -> [w936 _]
          frame False {
          }
          frame True {
            n545 = global read "Trav_pos_global.vi" "Current Row"() -> (w942:T17)
            n546 = Unbundle By Name(w942) -> ("Averaging time (min)"=w940:dbl)
            n547 = Multiply(x=60.0 ("y"), y=w940) -> (x*y=w938:dbl)
            n548 = Subtract(x=w939, y=w938) -> (x-y=w937:dbl)
          }
        }
        n549 = case shown="True" w931 {
          tunnel: w934 -> [_ _]
          tunnel: w920 -> [w945 w997]
          tunnel: w929 -> [w944 w996]
          tunnel: w919 -> [w943 w995]
          frame True {
            n550 = stacked-sequence {
              seq-local: [_ w949 _ _ _] -> [_ _ w955 _ _]
              seq-local: [_ _ _ w968 _] -> [_ _ _ _ w988]
              tunnel: w945 -> [w948 _ _ _ _]
              tunnel: w944 -> [w947 _ _ _ _]
              tunnel: w943 -> [w946 _ _ _ _]
              frame #0 {
                n551 = call "Write_Results_file.vi"("Experiment start time"=w946, "Experiment End time"=w948, "Setup filename"=w947) -> ()  [unwired: 4 out]
              }
              frame #1 {
                n552 = global read "Meas_global.vi" "Second Graph"() -> (w953:T3)
                n553 = global read "Meas_global.vi" "First Graph"() -> (w954:T3)
                n554 = Unbundle By Name(w953) -> ("Save graph"=w951:u16)
                n555 = Unbundle By Name(w954) -> ("Save graph"=w952:u16)
                n556 = Add(x=w952, y=w951) -> (x+y=w950:u16)
                n557 = Not Equal To 0?(x=w950) -> (x != 0?=w949:bool)
              }
              frame #2 {
                n558 = case shown="True" w955 {
                  frame False {
                  }
                  frame True {
                    n559 = stacked-sequence {
                      tunnel: "Show Smoth" -> [w959 w960]
                      frame #0 {
                        n560 = local read "First plot"() -> (w958:cluster{"Xo":dbl, "Delta X":dbl, dbl[]}[])
                        n561 = local read "2nd plot"() -> (w957:cluster{"Xo":dbl, "Delta X":dbl, dbl[]}[])
                        n562 = call "Save_plot_routine.vi"("Show Smooth"=w959, "First Plot data"=w958, "Second Plot data"=w957) -> ()  [unwired: 1 in, 3 out]
                      }
                      frame #1 {
                        n563 = case shown="True" w960 {
                          frame False {
                          }
                          frame True {
                            n564 = Open VI Reference(vi path="Measurement.vi") -> (vi reference=w966:refnum<vi>, error out=w962:errorcluster)  [unwired: 1 in, 4 out]
                            n565 = local write "Show Smoth"(FALSE ("Show Smoth")) -> ()
                            n566 = property class="VI"(reference=w966, error in=w962, "Front Panel Window:Is Frontmost"=TRUE) -> (reference out=w964:refnum<vi>, error out=w963:errorcluster)
                            n567 = Close Reference(reference=w964, error in (no error)=w963) -> ()  [unwired: 1 out]
                          }
                        }
                      }
                    }
                  }
                }
              }
              frame #3 {
                w973 = FALSE  # Empty list
                n568 = global read "Meas_global.vi" "Raw data file"() -> (w972:path)
                n569 = global read "Trav_pos_global.vi" "Top level setup filename"() -> (w970:path)
                n570 = global read "Meas_global.vi" "Start Time of experiment"() -> (w969:dbl)
                n571 = Strip Path(path=w972) -> (stripped path=w968:path)  [unwired: 1 out]
                n572 = Empty String/Path?(string/path=w970) -> (empty?=w971:bool)
                n573 = case shown="False" w971 {
                  tunnel: w970 -> [w987 _]
                  tunnel: w968 -> [w985 _]
                  tunnel: w969 -> [w983 _]
                  frame False {
                    n574 = call "Sec_to_date_filename.vi"("seconds"=w983) -> ("Day"=w982:string, "Time"=w981:string)  [unwired: 2 out]
                    n575 = Format Into String(format string="Cmd_%s_%s.xls", w982, w981) -> (resulting string=w979:string)  [unwired: 2 in, 1 out]
                    n576 = call "Fast_string_Replace.vi"("Replace match with:"="-", "Input String"=w979, "regular expression"=":") -> ("Output String"=w976:string)  [unwired: 2 out]
                    n577 = call "Fast_string_Replace.vi"("Replace match with:"="", "Input String"=w976, "regular expression"=" ") -> ("Output String"=w974:string)  [unwired: 2 out]
                    n578 = Build Path(base path=w985, name or relative path=w974) -> (appended path=w984:path)
                    n579 = Copy(10:w984, 11:w987) -> ()  [unwired: 1 in, 5 out]
                  }
                  frame True {
                  }
                }
                n580 = call "Remember_RD_Folders.vi"("Empty list"=w973, "Folders to Remember"=w968) -> ()  [unwired: 1 out]
              }
              frame #4 {
                n581 = global read "Meas_global.vi" "LDA data"() -> (w989:enum16{"No LDA data", "Take LDA data"})
                n582 = case shown="\"Take LDA data\"" w989 {
                  tunnel: w988 -> [_ w993]
                  frame "No LDA data" {
                  }
                  frame "Take LDA data" {
                    w991 = "LDA_Probe_Orientation.txt" ("name or relative path")
                    n583 = call "Setup_Filepath.vi"("Setup File Type"=Setup_Filetype."General", "Filename in"=w991) -> ("Filename Out"=w990:path)  [unwired: 1 out]
                    n584 = Build Path(base path=w993, name or relative path=w991) -> (appended path=w994:path)
                    n585 = Copy(10:w994, 11:w990) -> ()  [unwired: 1 in, 5 out]
                  }
                }
              }
            }
          }
          frame False {
            n586 = global read "Meas_global.vi" "Raw data option"() -> (w998:enum16{"Save raw data", "Raw data not saved"})
            n587 = case shown="\"Save raw data\"" w998 {
              tunnel: w995 -> [w1001 _]
              tunnel: w997 -> [w1000 _]
              tunnel: w996 -> [w999 _]
              frame "Save raw data" {
                n588 = stacked-sequence {
                  tunnel: w1001 -> [_ w1010]
                  tunnel: w1000 -> [_ w1009]
                  tunnel: w999 -> [_ w1007]
                  frame #0 {
                    n589 = global read "Meas_global.vi" "Current Block No"() -> (w1002:i32)
                    n590 = global write "Meas_global.vi" "Requested No of blocks"(w1002) -> ()
                  }
                  frame #1 {
                    n591 = call "Create_Raw_data_file.vi"("No of averages"=1, "End time"=w1009, "Start time"=w1010, "Setup filename"=w1007) -> ("Values"=w1005:string[][], "Column headers"=w1006:string[])  [unwired: 2 out]
                    n592 = Index Array(array=w1005, index (row)=0) -> (element=w1003:string[])  [unwired: 1 in]
                    n593 = global write "Dynamic_call_global.ph.vi" "Plug in values"(w1003) -> ()
                    n594 = global write "Dynamic_call_global.ph.vi" "Plug in titles"(w1006) -> ()
                  }
                }
              }
              frame "Raw data not saved" {
              }
            }
          }
        }
      }
      frame #19 {
        n595 = stacked-sequence {
          seq-local: [w1017 _] -> [_ w1026]
          seq-local: [w1013 _] -> [_ w1025]
          tunnel: w1011 -> [w1024 _]
          frame #0 {
            n596 = global read "Meas_global.vi" "Raw data file"() -> (w1015:path)
            n597 = global read "Meas_global.vi" "Raw data option"() -> (w1023:enum16{"Save raw data", "Raw data not saved"})
            n598 = Equal?(x=Setup."Run Program" ("setup"), y=w1024) -> (x = y?=w1019:bool)
            n599 = Strip Path(path=w1015) -> (stripped path=w1014:path)  [unwired: 1 out]
            n600 = Equal?(x=w1023, y=enum16{"Save raw data", "Raw data not saved"}."Save raw data" ("Raw data option")) -> (x = y?=w1018:bool)
            n601 = Build Path(base path=w1014, name or relative path="VI_History.xls") -> (appended path=w1013:path)
            n602 = call "Does_file_exist_(simple).vi"("Pathname"=w1013) -> ("exists?"=w1021:bool)
            n603 = Not(x=w1021) -> (.not. x?=w1020:bool)
            n604 = Compound Arithmetic op=AND(w1020, w1019, w1018) -> (w1017:bool)
          }
          frame #1 {
            n605 = case shown="True" w1026 {
              tunnel: w1025 -> [_ w1033]
              frame False {
              }
              frame True {
                w1027 = FALSE  # Lock File
                n606 = global read "Meas_global.vi" "Prog's last revision date"() -> (w1030:u32)
                n607 = Get Date/Time String(date format (0)=enum16{"short", "long", "abbreviated"}."abbreviated", seconds (now)=w1030) -> (date string=w1029:string)  [unwired: 2 out]
                n608 = call "Characters_to_string.vi"("Characters to write"=w1029, "Label for characters"="Prog's last revision date") -> ("Output string"=w1035:string)
                n609 = call "Date_and_Time_to_string.vi"() -> ("Date and time (spreadsheet)"=w1036:string)
                n610 = call "Get_mod_dates.vi"() -> ("error out"=w1034:errorcluster, "Output string"=w1028:string)  [unwired: 1 in, 3 out]
                n611 = call "EnFlo_Error_Handler.vi"("error in (no error)"=w1034) -> ()  [unwired: 2 in, 3 out]
                n612 = Concatenate Strings(w1036, w1035, w1028) -> (w1032:string)
                n613 = call "Write_Characters_To_File.vi"("file path (dialog if empty)"=w1033, "character string"=w1032, "Lock File"=w1027) -> ()  [unwired: 2 in, 4 out]
              }
            }
          }
        }
      }
      frame #20 {
        w1040 = FALSE ("Remote control")
        n614 = local read "Correlate?"() -> (w1042:T6)
        n615 = case shown="\"Run Program\"" w1039 {
          tunnel: w1039 -> [w1046 _ _ _]
          tunnel: [w1046 w1063 w1064 w1065] -> w1038
          frame "Run Program" {
            n616 = global read "Meas_global.vi" "Velocity Cluster Array"() -> (w1045:T27[])
            n617 = Array Size(array=w1045) -> (size(s)=w1044:i32)
            n618 = Decrement(x=w1044) -> (x-1=w1043:i32)
            n619 = while {
              tunnel: w1045 -> [w1061] mode=indexing
              tunnel: w1043 -> [w1052]
              i -> [w1053]
              stop <- w1050 continue-if-true
              w1058 = "Pitot ("
              n620 = Unbundle By Name(w1061) -> ("U"=w1047:dbl, "Name"=w1057:string)
              n621 = String Length(string=w1058) -> (length=w1060:i32)
              n622 = String Subset(string=w1057, length (rest)=w1060) -> (substring=w1059:string)  [unwired: 1 out]
              n623 = Equal?(x=w1059, y=w1058) -> (x = y?=w1054:bool)
              n624 = call "Match_Pat_Case_In.vi"("String to match"="ref", "String"=w1057) -> ("offset past match"=w1055:i32)  [unwired: 1 in, 3 out]
              n625 = Greater Or Equal To 0?(x=w1055) -> (x >= 0?=w1049:bool)
              n626 = Less?(x=w1053, y=w1052) -> (x < y?=w1051:bool)
              n627 = And(x=w1049, y=w1054) -> (x .and. y?=w1048:bool)
              n628 = case shown="True" w1048 {
                tunnel: w1047 -> [_ w1062]
                frame False {
                }
                frame True {
                  n629 = call "Log_Reference_Velocity.vi"("Measured Velocity"=w1062) -> ()  [unwired: 1 out]
                }
              }
              n630 = Compound Arithmetic op=AND(invert w1048, w1051) -> (w1050:bool)
            }
          }
          frame "Show Setup" {
            w1063 = Setup."Run Program"  # setup
          }
          frame "Save Current Setup" {
            w1064 = Setup."Run Program"  # setup
          }
          frame "Setup Front Panel" {
            w1065 = Setup."Run Program"  # setup
          }
        }
        n631 = case shown="\"Correlate without activating panel\"" w1042 {
          tunnel: [T6."Cross correlation off" T6."Correlate without activating panel" T6."Correlate without activating panel"] -> w1041
          frame "Cross correlation off" {
          }
          frame "Show correlation panel" {
          }
          frame "Correlate without activating panel" {
          }
        }
        n632 = local write "Correlate?"(w1041) -> ()
        n633 = global write "Meas_global.vi" "Remote control"(w1040) -> ()
        n634 = global write "Dynamic_call_global.ph.vi" "Acquisition Interlock"(w1040) -> ()
        n635 = call "Program_Active.vi"() -> ()  [unwired: 1 in]
        n636 = local write "setup"(w1038) -> ()
      }
      frame #21 {
        w1073 = FALSE  # Dialog Box (T)
        n637 = global read "Meas_global.vi" "Over/Under string"() -> (w1071:string)
        n638 = Empty String/Path?(string/path=w1071) -> (empty?=w1070:bool)
        n639 = Not(x=w1070) -> (.not. x?=w1069:bool)
        n640 = Bundle By Name(cluster=errorcluster {"status"=FALSE, "code"=0, "source"=""} ("error in (no error)"), "source"=w1071, "status"=w1069) -> (w1074:errorcluster)
        n641 = call "EnFlo_Error_Handler.vi"("error in (no error)"=w1074, "Error Type"="Signal Clipping", "Dialog Box (T)"=w1073) -> ()  [unwired: 3 out]
      }
      frame #22 {
        w1078 = string[] [] ("Per Block Plug Ins Extra")
        n642 = Empty String/Path?(string/path=w1082) -> (empty?=w1081:bool)
        n643 = global read "Dynamic_call_global.ph.vi" "Final Plug Ins"() -> (w1083:string[])
        n644 = case shown="True" w1081 {
          tunnel: w1082 -> [w1095 _]
          frame False {
            n645 = local read "Comments"() -> (w1094:string)
            n646 = call "Fast_string_Replace.vi"("Replace match with:"="", "Input String"=w1094, "regular expression"=w1095) -> ("Output String"=w1093:string)  [unwired: 2 out]
            n647 = local write "Comments"(w1093) -> ()
          }
          frame True {
          }
        }
        n648 = call "Plug_in_Directories.vi"() -> ("Final"=w1079:path)  [unwired: 3 out]
        n649 = for {
          tunnel: w1083 -> [w1098] mode=indexing
          tunnel: w1079 -> [w1097]
          w1101 = FALSE  # Dialog Box (T)
          n650 = Build Path(base path=w1097, name or relative path=w1098) -> (appended path=w1096:path)
          n651 = global read "Dynamic_call_global.ph.vi" "Plug in"() -> (w1106:refnum<vi>)
          n652 = Open VI Reference(type specifier VI Refnum (for type only)=w1106, vi path=w1096) -> (vi reference=w1105:refnum<vi>, error out=w1104:errorcluster)  [unwired: 2 in, 2 out]
          n653 = call-by-ref "?"(reference=w1105, error in=w1104) -> (reference out=w1102:refnum<vi>, error out=w1103:errorcluster)  [unwired: 6 in, 2 out]
          n654 = Close Reference(reference=w1102, error in (no error)=w1103) -> (error out=w1099:errorcluster)
          n655 = call "EnFlo_Error_Handler.vi"("error in (no error)"=w1099, "Error Type"="Running Final Plug In", "Dialog Box (T)"=w1101) -> ()  [unwired: 3 out]
        }
        n656 = global read "Meas_global.vi" "Repeat Measurement?"() -> (w1080:bool)
        n657 = case shown="False" w1080 {
          tunnel: w1077 -> [_ w1091]
          tunnel: [FALSE w1086] -> w1076
          frame False {
            n658 = global write "Trav_pos_global.vi" "Present Probe Positions"(T7 [] ("Present Probe Positions")) -> ()
          }
          frame True {
            n659 = global read "Meas_global.vi" "Post Process"() -> (w1089:T5)
            n660 = Equal To 0?(x=w1091) -> (x = 0?=w1087:bool)
            n661 = Equal?(x=w1089, y=Post_Process."Post Process Raw Data File" ("Post Process")) -> (x = y?=w1088:bool)
            n662 = And(x=w1088, y=w1087) -> (x .and. y?=w1086:bool)
          }
        }
        n663 = global write "Dynamic_call_global.ph.vi" "Per Block Plug Ins Extra"(w1078) -> ()
        n664 = global write "Dynamic_call_global.ph.vi" "Initial Plug Ins Extra"(w1078) -> ()
      }
      frame #23 {
        n665 = global read "Meas_global.vi" "Post Process"() -> (w1113:T5)
        n666 = local read "stop"() -> (w1119:bool)
        n667 = Equal?(x=w1114, y=Setup."Run Program" ("setup")) -> (x = y?=w1110:bool)
        n668 = Equal?(x=w1113, y=Post_Process."Take New Data" ("Post Process")) -> (x = y?=w1111:bool)
        n669 = And(x=w1110, y=w1111) -> (x .and. y?=w1109:bool)
        n670 = case shown="False" w1119 {
          tunnel: [Multi_Run_Status."Continue" ("Status Out") Multi_Run_Status."Terminate Run" ("Status Out")] -> w1117
          frame False {
          }
          frame True {
            n671 = local write "stop"(FALSE) -> ()
          }
        }
        n672 = case shown="True" w1109 {
          tunnel: w1117 -> [w1120 w1123]
          tunnel: [w1120 w1125] -> w1116
          frame False {
          }
          frame True {
            n673 = local read "Raw data file"() -> (w1124:path)
            n674 = Path to Array of Strings(0:w1124) -> (2:w1126:string[])  [unwired: 1 out]
            n675 = Index Array(array=w1126, index=0 ("Index")) -> (element=w1122:string)
            n676 = Build Array(w1122) -> (w1121:string[])
            n677 = for {
              tunnel: w1121 -> [w1130] mode=indexing
              shift-right: [w1128] -> w1125
              shift-left: w1123 -> [w1129]
              n678 = call "Warn_on_low_HD_space.vi"("Status In"=w1129, "HD name"=w1130) -> ("Status Out"=w1128:T4)  [unwired: 6 out]
            }
          }
        }
        "Status Out" <- w1116
        n679 = global write "Trav_pos_global.vi" "Dummy Measurement?"(FALSE ("Dummy Measurement?")) -> ()
        n680 = global write "Plug_in_data_global.vi" "Server Channels to log"(string[] [] ("Server Channels to log")) -> ()
        n681 = global write "Meas_global.vi" "Extra Comments"("") -> ()
      }
    }
  }
